vi "EC_Applied_Motion_SXSYSZ_20170419_3ch.vi"() -> ()   [LabVIEW 2015]
uses:
  <vilib>/Utility/file.llb/Read From Spreadsheet File (I64).vi
  <vilib>/Utility/file.llb/Read From Spreadsheet File (string).vi
  <vilib>/Instr/_visa.llb/VISA Configure Serial Port (Instr).vi
  <vilib>/Utility/file.llb/Write To Spreadsheet File (I64).vi
  <vilib>/Utility/file.llb/Write To Spreadsheet File (string).vi
panel:
  in  "Cancel Button":bool
  in  "APX:FZ_JN":bool
  in  "APX:FZ_JP":bool
  in  "APX:FY_JN":bool
  in  "APX:FY_JP":bool
  in  "APX:FX_JN":bool
  in  "APX:FX_JP":bool
  out "Z Velocity MV mm/sec":dbl format="%.3f"
  out "Z Position MV mm":dbl
  out "Y Velocity MV mm/sec":dbl format="%.3f"
  out "Y Position MV mm":dbl
  out "X Velocity MV mm/sec":dbl format="%.3f"
  out "X Position MV mm":dbl
  out "Presets":i32[][](array[numeric])
  in  "stop":bool
  in  "Tab Control 3":enum32{"Status", "Reset"}(tab)
  out "Y in Range":bool
  out "Y Scan":bool
  out "Y in Motion":bool
  out "Y Backlash corr":bool
  out "X  in Range":bool
  out "X Scan":bool
  out "X  in Motion":bool
  out "X Backlash corr":bool
  out "Z in Range":bool
  out "Z Scan":bool
  out "Z in Motion":bool
  out "Z Backlash corr":bool
  out "X Ready":bool
  out "Y Ready":bool
  out "Z Ready":bool
  in  "Reset Y Position mm":dbl
  out "Reset Y Motor Steps":i32
  in  "Reset X Position mm":dbl
  out "Reset X Motor Steps":i32
  in  "Reset Z Position mm":dbl
  out "Reset Z Motor Steps":i32
  in  "Reset":bool
  in  "Tab Control 2":enum32{"mm", "step"}(tab)
  in  "X Scan Length SP mm":dbl
  in  "X Scan Velocity SP mm/sec":dbl
  in  "X Scan set":bool
  in  "Y Scan Length SP mm":dbl
  in  "Y Scan Velocity SP mm/sec":dbl
  in  "Y Scan set":bool
  in  "Z Scan Length SP mm":dbl
  in  "Z Scan Velocity SP mm/sec":dbl
  in  "Z Scan set":bool
  in  "X Scan Velocity SP steps/sec":i32=1 min=1 max=102400 step=1
  in  "X Scan Length SP steps":i32 min=-500000 max=500000 step=100
  out "X Scan length MV mm":dbl
  out "X Scan velocity MV mm/sec":dbl format="%#_6f"
  in  "Y Scan Velocity SP steps/sec":i32=1 min=1 max=102400 step=1
  in  "Y Scan Length SP steps":i32 min=-1000000 max=0 step=100
  out "Y Scan length MV mm":dbl
  out "Y Scan velocity MV mm/sec":dbl format="%#_6f"
  in  "Z Scan Velocity SP steps/sec":i32=1 min=1 max=102400 step=1
  in  "Z Scan Length SP steps":i32 min=-204724 max=102195276 step=100
  out "Z Scan length MV mm":dbl
  out "Z Scan velocity MV mm/sec":dbl format="%#_6f"
  out "atan Y/Z":dbl
  in  "Tab Control":enum32{"mm", "preset", "step"}(tab)
  in  "X Position SP mm":dbl
  in  "X Velocity SP mm/sec":dbl=0.01
  in  "X Move Set":bool
  in  "Y Move Set":bool
  in  "Y Position SP mm":dbl
  in  "Y Velocity SP mm/sec":dbl=0.01
  in  "Z Position SP mm":dbl
  in  "Z Velocity SP mm/sec":dbl=0.05
  in  "Z Move Set":bool
  in  "Add Button":bool
  in  "String":string
  in  "Delete Button":bool
  in  "Preset positions":i32(ring) items=["ZERO", "Default", "CDOSE", "QMS", "test", "test2", "test3"]
  in  "Set Button":bool
  in  "X Velocity SP step/sec":i32 min=1 max=100
  in  "Y Velocity SP step/sec":i32 min=1 max=100
  in  "Z Velocity SP step/sec":i32 min=1 max=50
  in  "Y Step SP":i32=-20000 min=-800000 max=800000 step=500
  in  "X Step SP":i32=-20000 min=-750000 max=750000 step=500
  in  "Z Step SP":i32=-20000 min=-3000 max=102400000 step=500
  out "X Step PV":i32 max=2000
  out "Y Step PV":i32 max=2000
  out "Z Step PV":i32 max=2000
  out "R Step PV":i32 max=2000
  out "X Scan Duration":dbl
  out "Y Scan Duration":dbl
  out "Z Scan Duration":dbl
  out "Z COM PORT":refnum<visa-resource-name>="COM5"
  out "Z Backlash steps/sec":i32
  out "Z Backlash":i32
  out "Z Holding Current %":i32
  out "Z Run Current %":i32
  out "Z offset mm":dbl
  out "Z mm/rev":dbl
  out "Z steps/rev":u32
  out "Z  velocity PV step/sec":i32
  out "Z MINPOS":i32=-94296
  out "Z MAXPOS":i32=-34296
  in  "Z Scan OK":bool
  in  "Z Go":bool
  out "Z Position mm PV":dbl
  out "X Position mm PV":dbl
  out "X velocity PV step/sec":i32
  in  "X Scan OK":bool
  in  "X Go":bool
  out "X Backlash steps/sec":i32
  out "X Backlash":i32
  out "X Holding Current %":i32
  out "X Run Current %":i32
  out "X offset mm":dbl
  out "X mm/rev":dbl
  out "X steps/rev":u32
  out "X MAXPOS":i32=-34296
  out "X MINPOS":i32=-94296
  out "X COM PORT":refnum<visa-resource-name>="COM5"
  out "Y Backlash steps/sec":i32
  out "Y Backlash":i32
  out "Y Holding Current %":i32
  out "Y Run Current %":i32
  in  "Scan Cancel":bool
  out "Y Position mm PV":dbl
  out "Y offset mm":dbl
  out "Y mm/rev":dbl
  out "Y steps/rev":u32
  out "Y velocity PV step/sec":i32
  in  "Y Scan OK":bool
  in  "Scan Go":bool
  in  "Stop":bool
  in  "Y Go":bool
  out "Y MINPOS":i32=-94296
  out "Y MAXPOS":i32=-34296
  out "Y COM PORT":refnum<visa-resource-name>="COM5"
  # "APX:FinePos"
  # "Current position"
  # "Goto position"
  # "APX:FX"
  # "FX"
  # "APX:FY"
  # "FY"
  # "FZ"
  # "APX:FZ"
  # "R,L = green"
  # "L"
  # "M"
  # "B"
  # "S"
  # "R"
  # "Preset position"
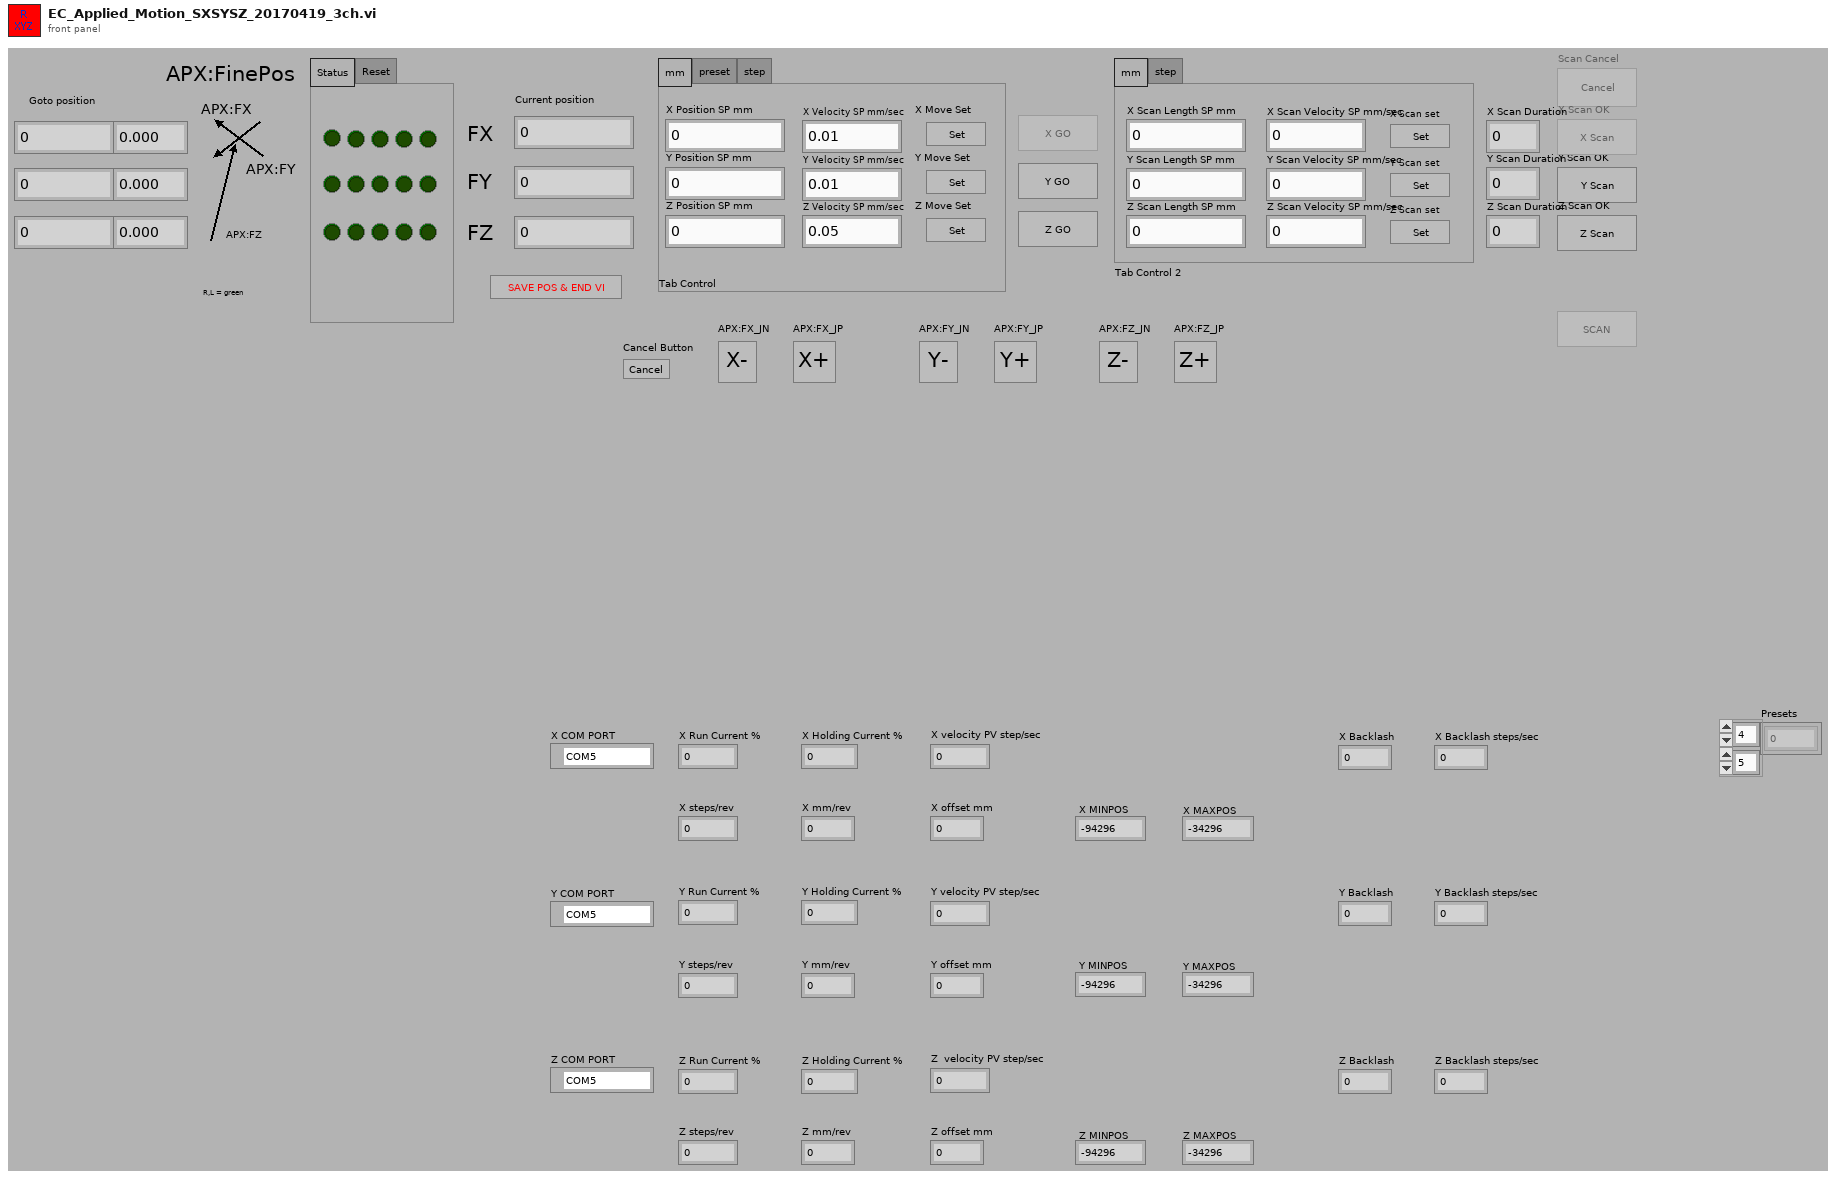
[diagram p1: front panel]
types:
  T1 = enum16{"Power-up Signature", "Accel Rate", "Accel Max", "Bit Rate", "Buffer Status", "Change Current", "Commence Jogging", "Change Jog Speed", "Continue", "Define Address", "Distance for FC,FM,FO,FY", "Decel Rate", "Distance or Position", "Define Limits", "Encoder Deadband", "Encoder Function", "Encoder Position", "Encoder Ratio", "Feed to Length with Speed Change", "Feed to Length", "Feed to Sensor with Mask Dist", "Feed to Length & Set Output", "Feed to Position", "Feed to Sensor", "Feed to Sensor w/safety", "Follow Handwheel", "Immediate Distance?", "Immediate Encoder?", "Immediate Low Output", "Immediate High Output", "Immediate Position?", "Input Status?", "Jog Accel/Decel", "Jog Disable", "Jog Enable", "Jog Speed", "Motor Disable", "Motor Enable", "Microstep Resolution", "Power up Current", "Power up Mode", "Pause", "Request Status", "Revision Level?", "Seek Home", "Stop Jogging", "Stop & Kill Buffer", "Set Output", "Set ABS Position", "Send String", "Stop", "Velocity for Speed Change", "Velocity Setting", "Wait for Input", "Wait Time"}
  T2 = enum8{"Enabled", "Disabled", "Disabled and Grayed Out"}
  T3 = cluster{"first row[0]":i64, "first row[1]":i64, "first row[2]":i64, "first row[3]":i64, "first row[4]":i64, "first row[5]":i64, "first row[6]":i64, "first row[7]":i64, "first row[8]":i64}
  T4 = cluster{"Value[0]":i32, "Value[1]":i32, "Value[2]":i32, "Value[3]":i32, "Value[4]":i32, "Value[5]":i32, "Value[6]":i32, "Value[7]":i32, "Value[8]":i32}
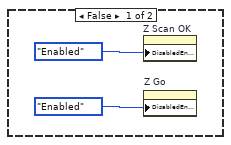
[diagram p5: hidden frame]
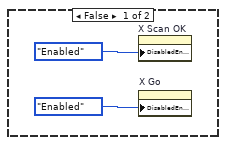
[diagram p9: hidden frame]
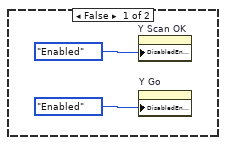
[diagram p13: hidden frame]
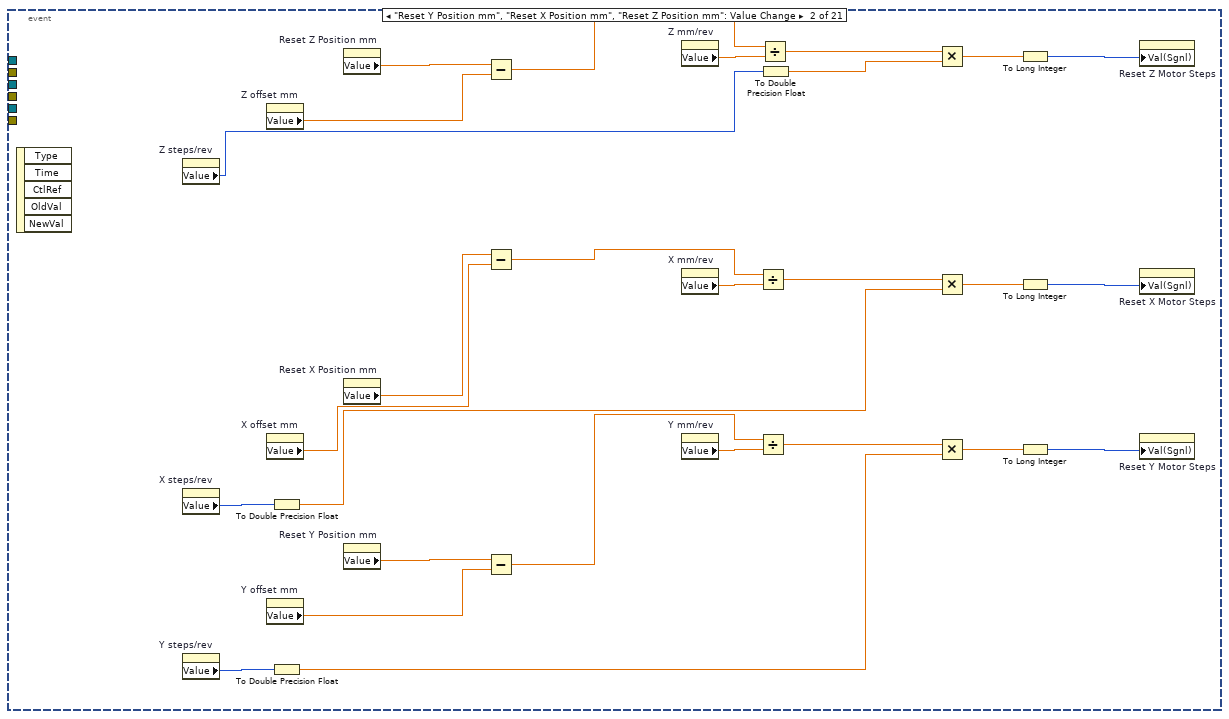
[diagram p17: hidden frame]
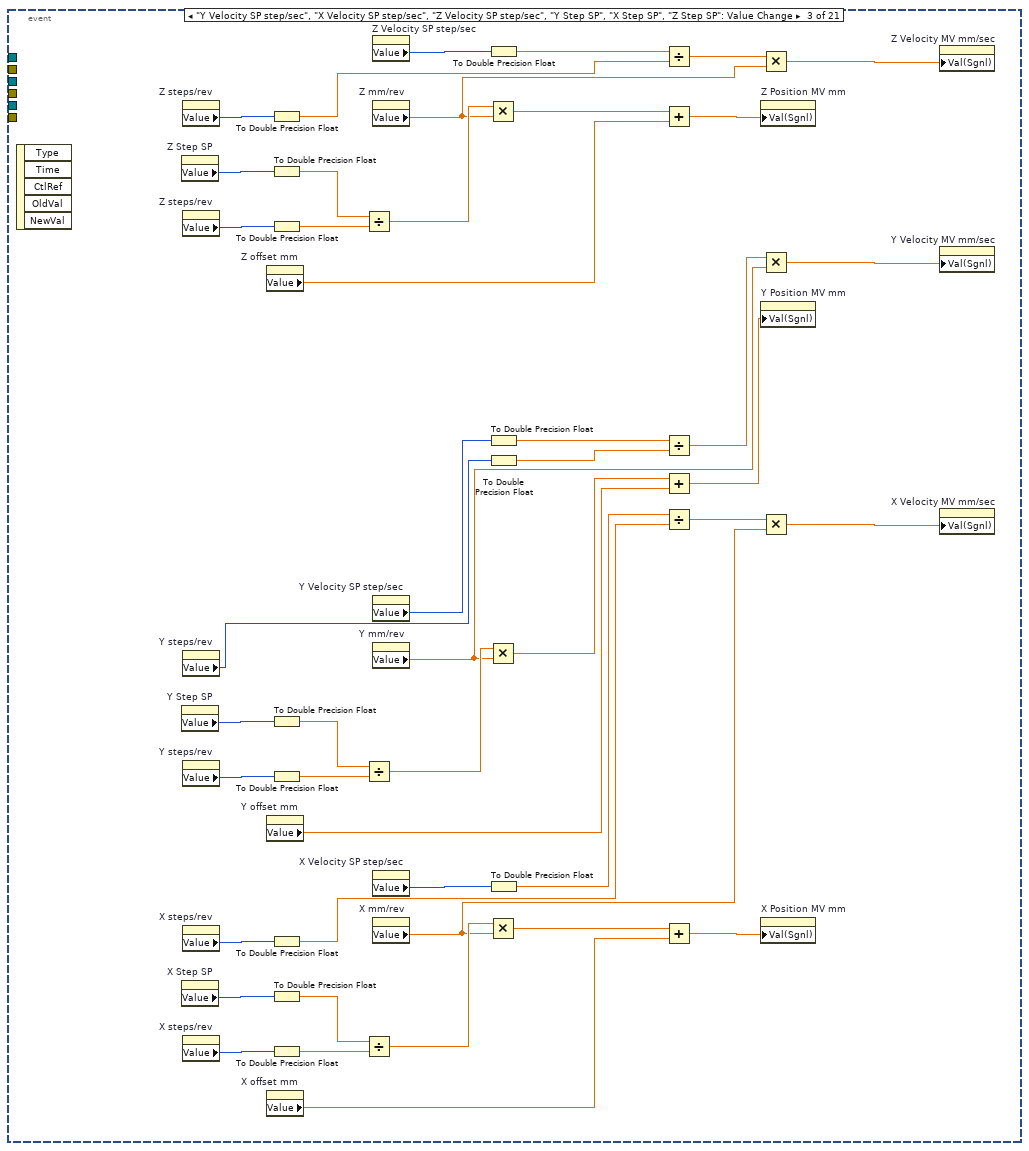
[diagram p18: hidden frame]
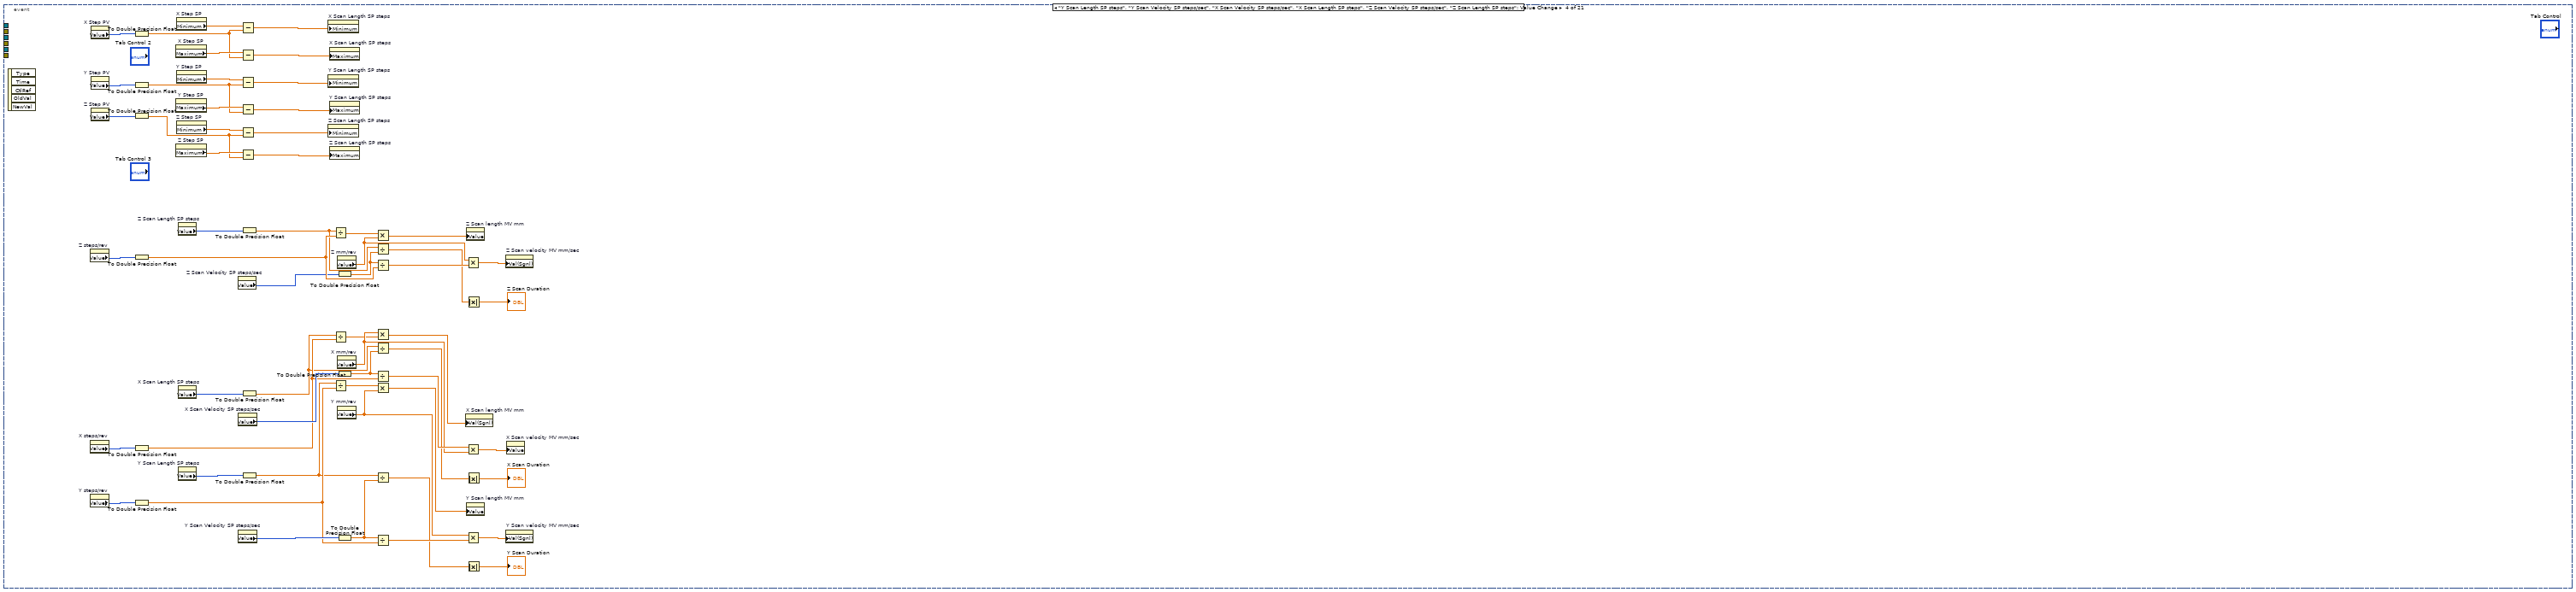
[diagram p19: hidden frame]
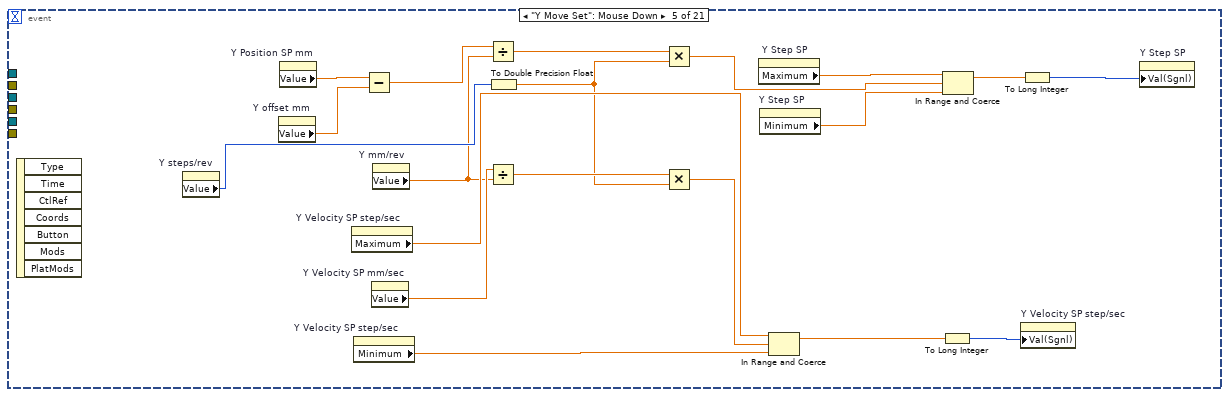
[diagram p20: hidden frame]
diagram:
  (unwired) FALSE
  w19 = 0 ("dimension size")
  n1 = flat-sequence {
    tunnel: [w78] -> w5
    tunnel: [w77] -> w4
    tunnel: w5 -> [w92]
    tunnel: w4 -> [w91]
    tunnel: [w90] -> w3
    tunnel: [w89] -> w2
    tunnel: [w100] -> w49
    tunnel: [w99] -> w48
    tunnel: w3 -> [w102]
    tunnel: w2 -> [w101]
    tunnel: w49 -> [w117]
    tunnel: w48 -> [w116]
    tunnel: [w118] -> w47
    tunnel: [w119] -> w46
    tunnel: [w120] -> w1
    tunnel: [w131] -> w44
    tunnel: [w132] -> w45
    tunnel: w47 -> [w132]
    tunnel: w46 -> [w131]
    tunnel: w1 -> [w129]
    frame #0 {
      "Z Run Current %" <- 100 ("Z Run Current %")
      "Z Holding Current %" <- 50 ("Z Holding Current %")
    }
    frame #1 {
      "Z Backlash steps/sec" <- 1000 ("Z Backlash steps/sec")
      "Z Backlash" <- -2500 ("Z Backlash")
    }
    frame #2 {
      w68 = 2.54 ("Z mm/rev")
      w67 = u32 20000 ("step/rev")
      w69 = 50 ("Value (Signaling)")
      n2 = property on="Z Velocity SP step/sec" class="DigNum (strict)"("Minimum"=1.0 ("Data Entry Limits:Minimum")) -> ()  [unwired: 2 in, 2 out]
      n3 = property on="Z Scan Velocity SP mm/sec" class="DigNum (strict)"("Val(Sgnl)"=0.05 ("Value (Signaling)")) -> ()  [unwired: 2 in, 2 out]
      n4 = property on="Z Velocity SP step/sec" class="DigNum (strict)"("Val(Sgnl)"=w69) -> ()  [unwired: 2 in, 2 out]
      n5 = To Double Precision Float(number=w69) -> (double precision float=w73:dbl)
      n6 = property on="Z Velocity SP step/sec" class="DigNum (strict)"("Maximum"=w73) -> ()  [unwired: 2 in, 2 out]
      n7 = To Double Precision Float(number=w67) -> (double precision float=w72:dbl)
      n8 = Divide(x=w73, y=w72) -> (x/y=w70:dbl)
      n9 = Multiply(x=w70, y=w68) -> (x*y=w71:dbl)
      n10 = property on="Z Velocity SP mm/sec" class="DigNum (strict)"("Val(Sgnl)"=w71) -> ()  [unwired: 2 in, 2 out]
      "Z mm/rev" <- w68
      "Z steps/rev" <- w67
    }
    frame #3 {
      w75 = -3000 ("lower limit")
      w74 = 102400000 ("upper limit")
      n11 = property on="Z Step SP" class="DigNum (strict)"("Minimum"=w75) -> ()  [unwired: 2 in, 2 out]
      n12 = property on="Z Step SP" class="DigNum (strict)"("Maximum"=w74) -> ()  [unwired: 2 in, 2 out]
      "Z offset mm" <- 0.0 ("Z offset mm")
      "Z MINPOS" <- w75
      "Z MAXPOS" <- w74
    }
    frame #4 {
      w85 = refnum<visa-resource-name> "COM23" ("COM PORT")
      w83 = u16 0 items=["None", "XON/XOFF", "RTS/CTS", "XON/XOFF & RTS/CTS", "DTR/DSR", "XON/XOFF & DTR/DSR"] ("flow control (0:none)")
      w82 = u16 10 items=["1.0"=10, "1.5"=15, "2.0"=20] ("stop bits (10: 1 bit)")
      # "Stop bits"
      n13 = call-poly "VISA Configure Serial Port"("VISA resource name"=w85, "timeout (10sec)"=u32 10000, "baud rate (9600)"=u32 9600, "data bits (8)"=u16 8, "parity (0:none)"=enum16{"None", "Odd", "Even", "Mark", "Space"}."None", "stop bits (10: 1 bit)"=w82, "flow control (0:none)"=w83) -> ("VISA resource name out"=w78:refnum<visa-resource-name>, "error out"=w77:errorcluster)  [unwired: 7 in]
      "Z COM PORT" <- w85
    }
    frame #5 {
      # "Run Current %"
      n14 = property on="Z Run Current %" class="DigNum (strict)"() -> ("Value"=w93:i32)  [unwired: 2 in, 2 out]
      n15 = Divide(x=w93, y=100) -> (x/y=w94:dbl)
      n16 = Multiply(x=w94, y=3.5) -> (x*y=w88:dbl)
      n17 = Number To Fractional String(number=w88) -> (F-format string=w95:string)  [unwired: 3 in]
      n18 = call "Applied Send Command.vi"("error in (no error)"=w91, "Extra"=w95, "Command"=T1."Change Current", "VISA resource name"=w92) -> ("error out"=w89:errorcluster, "VISA resource name out"=w90:refnum<visa-resource-name>)  [unwired: 3 in, 1 out]
    }
    frame #6 {
      # "VELOCITY"
      n19 = property on="Z steps/rev" class="DigNum (strict)"() -> ("Value"=w98:u32)  [unwired: 2 in, 2 out]
      n20 = property on="Z Velocity SP step/sec" class="DigNum (strict)"() -> ("Value"=w97:i32)  [unwired: 2 in, 2 out]
      n21 = Divide(x=w97, y=w98) -> (x/y=w105:dbl)
      n22 = Number To Fractional String(number=w105) -> (F-format string=w107:string)  [unwired: 3 in]
      n23 = call "Applied Send Command.vi"("error in (no error)"=w101, "Extra"=w107, "Command"=T1."Velocity Setting", "VISA resource name"=w102) -> ("error out"=w108:errorcluster, "VISA resource name out"=w115:refnum<visa-resource-name>)  [unwired: 3 in, 1 out]
      n24 = call "Time Delay2"("error in (no error)"=w108, "Delay Time (s)"=0.1) -> ("error out"=w113:errorcluster)  [unwired: 9 in]
      n25 = call "Applied Send Command.vi"("error in (no error)"=w113, "Extra"="", "Command"=T1."Velocity Setting", "VISA resource name"=w115) -> ("error out"=w99:errorcluster, "read buffer"=w111:string, "VISA resource name out"=w100:refnum<visa-resource-name>)  [unwired: 3 in]
      n26 = Fract/Exp String To Number(string=w111, offset=3) -> (number=w106:dbl)  [unwired: 2 in, 1 out]
      n27 = Multiply(x=w106, y=w98) -> (x*y=w103:dbl)
      n28 = property on="Z  velocity PV step/sec" class="DigNum (strict)"("Val(Sgnl)"=w103) -> ()  [unwired: 2 in, 2 out]
    }
    frame #7 {
      # "GET CURRENT POSITION"
      n29 = call "Applied Send Command.vi"("error in (no error)"=w116, "Extra"="", "Command"=T1."Immediate Position?", "VISA resource name"=w117) -> ("error out"=w122:errorcluster, "read buffer"=w124:string, "VISA resource name out"=w118:refnum<visa-resource-name>)  [unwired: 3 in]
      n30 = call "Time Delay8"("error in (no error)"=w122, "Delay Time (s)"=0.1) -> ("error out"=w119:errorcluster)  [unwired: 9 in]
      n31 = Hexadecimal String To Number(string=w124, offset=3) -> (number=w120:u32)  [unwired: 1 in, 1 out]
    }
    frame #8 {
      n32 = property on="Z Step SP" class="DigNum (strict)"() -> ("Maximum"=w128:dbl)  [unwired: 2 in, 2 out]
      n33 = property on="Z Step SP" class="DigNum (strict)"() -> ("Minimum"=w127:dbl)  [unwired: 2 in, 2 out]
      n34 = property on="Z Step SP" class="DigNum (strict)"("Val(Sgnl)"=w129) -> ()  [unwired: 2 in, 2 out]
      n35 = In Range and Coerce(upper limit=w128, x=w129, lower limit=w127) -> (In Range?=w130:bool)  [unwired: 1 out]
      n36 = property on="Z in Range" class="Bool (strict)"("Val(Sgnl)"=w130) -> ()  [unwired: 2 in, 2 out]
    }
  }
  n37 = flat-sequence {
    frame #0 {
      n38 = property on="X Scan" class="Bool (strict)"("Val(Sgnl)"=FALSE ("Value (Signaling)")) -> ()  [unwired: 2 in, 2 out]
      n39 = property on="Y Scan" class="Bool (strict)"("Val(Sgnl)"=FALSE ("Value (Signaling)")) -> ()  [unwired: 2 in, 2 out]
      n40 = property on="Z Scan" class="Bool (strict)"("Val(Sgnl)"=FALSE ("Value (Signaling)")) -> ()  [unwired: 2 in, 2 out]
      n41 = property on="Scan Go" class="Bool"("DisabledEnum"=T2."Disabled and Grayed Out" ("Disabled")) -> ()  [unwired: 2 in, 2 out]
      n42 = property on="Scan Cancel" class="Bool"("DisabledEnum"=T2."Disabled and Grayed Out" ("Disabled")) -> ()  [unwired: 2 in, 2 out]
    }
    frame #1 {
      n43 = property on="Y Backlash corr" class="Bool (strict)"("Val(Sgnl)"=FALSE ("Value (Signaling)")) -> ()  [unwired: 2 in, 2 out]
      n44 = property on="X Backlash corr" class="Bool (strict)"("Val(Sgnl)"=FALSE ("Value (Signaling)")) -> ()  [unwired: 2 in, 2 out]
      n45 = property on="Z Backlash corr" class="Bool (strict)"("Val(Sgnl)"=FALSE ("Value (Signaling)")) -> ()  [unwired: 2 in, 2 out]
    }
  }
  n46 = flat-sequence {
    tunnel: [w158] -> w13
    tunnel: [w157] -> w12
    tunnel: w13 -> [w172]
    tunnel: w12 -> [w171]
    tunnel: [w170] -> w11
    tunnel: [w169] -> w10
    tunnel: w11 -> [w180]
    tunnel: w10 -> [w179]
    tunnel: [w178] -> w9
    tunnel: [w177] -> w8
    tunnel: [w197] -> w53
    tunnel: w9 -> [w200]
    tunnel: w8 -> [w199]
    tunnel: [w198] -> w7
    tunnel: [w196] -> w6
    tunnel: [w209] -> w59
    tunnel: [w212] -> w60
    tunnel: w53 -> [w209]
    tunnel: w7 -> [w212]
    tunnel: w6 -> [w210]
    frame #0 {
      "Y Run Current %" <- 100 ("Run Current %")
      "Y Holding Current %" <- 50 ("Holding Current %")
    }
    frame #1 {
      "Y Backlash" <- 5000 ("Backlash2")
      "Y Backlash steps/sec" <- 10000 ("Value (Signaling)")
    }
    frame #2 {
      w148 = 0.21167 ("MM/rev")
      w151 = u32 20000 ("step/rev")
      w146 = 100 ("Value (Signaling)")
      n47 = property on="Y Velocity SP step/sec" class="DigNum (strict)"("Minimum"=1.0 ("Data Entry Limits:Minimum")) -> ()  [unwired: 2 in, 2 out]
      n48 = property on="Y Scan Velocity SP mm/sec" class="DigNum (strict)"("Val(Sgnl)"=0.01 ("Value (Signaling)")) -> ()  [unwired: 2 in, 2 out]
      n49 = property on="Y Velocity SP step/sec" class="DigNum (strict)"("Val(Sgnl)"=w146) -> ()  [unwired: 2 in, 2 out]
      n50 = To Double Precision Float(number=w146) -> (double precision float=w152:dbl)
      n51 = property on="Y Velocity SP step/sec" class="DigNum (strict)"("Maximum"=w152) -> ()  [unwired: 2 in, 2 out]
      n52 = To Double Precision Float(number=w151) -> (double precision float=w150:dbl)
      n53 = Divide(x=w152, y=w150) -> (x/y=w147:dbl)
      n54 = Multiply(x=w147, y=w148) -> (x*y=w149:dbl)
      n55 = property on="Y Velocity SP mm/sec" class="DigNum (strict)"("Val(Sgnl)"=w149) -> ()  [unwired: 2 in, 2 out]
      "Y steps/rev" <- w151
      "Y mm/rev" <- w148
    }
    frame #3 {
      w155 = -800000 ("lower limit")
      w156 = 800000 ("upper limit")
      n56 = property on="Y Step SP" class="DigNum (strict)"("Minimum"=w155) -> ()  [unwired: 2 in, 2 out]
      n57 = property on="Y Step SP" class="DigNum (strict)"("Maximum"=w156) -> ()  [unwired: 2 in, 2 out]
      "Y MAXPOS" <- w156
      "Y MINPOS" <- w155
      "Y offset mm" <- 0.0 ("offset")
    }
    frame #4 {
      w165 = refnum<visa-resource-name> "COM22" ("COM PORT")
      w163 = u16 0 items=["None", "XON/XOFF", "RTS/CTS", "XON/XOFF & RTS/CTS", "DTR/DSR", "XON/XOFF & DTR/DSR"] ("flow control (0:none)")
      w162 = u16 10 items=["1.0"=10, "1.5"=15, "2.0"=20] ("stop bits (10: 1 bit)")
      # "Stop bits"
      n58 = call-poly "VISA Configure Serial Port"("VISA resource name"=w165, "timeout (10sec)"=u32 10000, "baud rate (9600)"=u32 9600, "data bits (8)"=u16 8, "parity (0:none)"=enum16{"None", "Odd", "Even", "Mark", "Space"}."None", "stop bits (10: 1 bit)"=w162, "flow control (0:none)"=w163) -> ("VISA resource name out"=w158:refnum<visa-resource-name>, "error out"=w157:errorcluster)  [unwired: 7 in]
      "Y COM PORT" <- w165
    }
    frame #5 {
      n59 = property on="Y Run Current %" class="DigNum (strict)"() -> ("Value"=w173:i32)  [unwired: 2 in, 2 out]
      n60 = Divide(x=w173, y=100) -> (x/y=w174:dbl)
      n61 = Multiply(x=w174, y=3.5) -> (x*y=w168:dbl)
      n62 = Number To Fractional String(number=w168) -> (F-format string=w175:string)  [unwired: 3 in]
      n63 = call "Applied Send Command.vi"("error in (no error)"=w171, "Extra"=w175, "Command"=T1."Change Current", "VISA resource name"=w172) -> ("error out"=w169:errorcluster, "VISA resource name out"=w170:refnum<visa-resource-name>)  [unwired: 3 in, 1 out]
    }
    frame #6 {
      # "VELOCITY"
      n64 = property on="Y steps/rev" class="DigNum (strict)"() -> ("Value"=w184:u32)  [unwired: 2 in, 2 out]
      n65 = property on="Y Velocity SP step/sec" class="DigNum (strict)"() -> ("Value"=w181:i32)  [unwired: 2 in, 2 out]
      n66 = Divide(x=w181, y=w184) -> (x/y=w183:dbl)
      n67 = Number To Fractional String(number=w183) -> (F-format string=w187:string)  [unwired: 3 in]
      n68 = call "Applied Send Command.vi"("error in (no error)"=w179, "Extra"=w187, "Command"=T1."Velocity Setting", "VISA resource name"=w180) -> ("error out"=w188:errorcluster, "VISA resource name out"=w195:refnum<visa-resource-name>)  [unwired: 3 in, 1 out]
      n69 = call "Time Delay36"("error in (no error)"=w188, "Delay Time (s)"=0.1) -> ("error out"=w193:errorcluster)  [unwired: 9 in]
      n70 = call "Applied Send Command.vi"("error in (no error)"=w193, "Extra"="", "Command"=T1."Velocity Setting", "VISA resource name"=w195) -> ("error out"=w177:errorcluster, "read buffer"=w191:string, "VISA resource name out"=w178:refnum<visa-resource-name>)  [unwired: 3 in]
      n71 = Fract/Exp String To Number(string=w191, offset=3) -> (number=w186:dbl)  [unwired: 2 in, 1 out]
      n72 = Multiply(x=w186, y=w184) -> (x*y=w185:dbl)
      n73 = property on="Y velocity PV step/sec" class="DigNum (strict)"("Val(Sgnl)"=w185) -> ()  [unwired: 2 in, 2 out]
    }
    frame #7 {
      # "GET CURRENT POSITION"
      n74 = call "Applied Send Command.vi"("error in (no error)"=w199, "Extra"="", "Command"=T1."Immediate Position?", "VISA resource name"=w200) -> ("error out"=w202:errorcluster, "read buffer"=w204:string, "VISA resource name out"=w198:refnum<visa-resource-name>)  [unwired: 3 in]
      n75 = call "Time Delay37"("error in (no error)"=w202, "Delay Time (s)"=0.1) -> ("error out"=w197:errorcluster)  [unwired: 9 in]
      n76 = Hexadecimal String To Number(string=w204, offset=3) -> (number=w196:u32)  [unwired: 1 in, 1 out]
    }
    frame #8 {
      n77 = property on="Y Step SP" class="DigNum (strict)"() -> ("Maximum"=w208:dbl)  [unwired: 2 in, 2 out]
      n78 = property on="Y Step SP" class="DigNum (strict)"() -> ("Minimum"=w207:dbl)  [unwired: 2 in, 2 out]
      n79 = property on="Y Step SP" class="DigNum (strict)"("Val(Sgnl)"=w210) -> ()  [unwired: 2 in, 2 out]
      n80 = In Range and Coerce(upper limit=w208, x=w210, lower limit=w207) -> (In Range?=w211:bool)  [unwired: 1 out]
      n81 = property on="Y in Range" class="Bool (strict)"("Val(Sgnl)"=w211) -> ()  [unwired: 2 in, 2 out]
    }
  }
  n82 = flat-sequence {
    tunnel: [w230] -> w18
    tunnel: [w229] -> w17
    tunnel: w18 -> [w247]
    tunnel: w17 -> [w246]
    tunnel: [w245] -> w16
    tunnel: [w244] -> w15
    tunnel: [w250] -> w58
    tunnel: w16 -> [w258]
    tunnel: w15 -> [w257]
    tunnel: [w251] -> w14
    tunnel: w58 -> [w272]
    tunnel: [w271] -> w52
    tunnel: [w269] -> w51
    tunnel: [w274] -> w50
    tunnel: w14 -> [w273]
    tunnel: [w283] -> w56
    tunnel: [w284] -> w57
    tunnel: w52 -> [w284]
    tunnel: w51 -> [w283]
    tunnel: w50 -> [w279]
    frame #0 {
      "X Run Current %" <- 100 ("Run Current %")
      "X Holding Current %" <- 50 ("Holding Current %")
    }
    frame #1 {
      "X Backlash steps/sec" <- 10000 ("Value (Signaling)")
      "X Backlash" <- 5000 ("Backlash2")
    }
    frame #2 {
      w219 = 0.21167 ("MM/rev")
      w222 = u32 20000 ("step/rev")
      w217 = 100 ("Value (Signaling)")
      n83 = property on="X Velocity SP step/sec" class="DigNum (strict)"("Minimum"=1.0 ("Data Entry Limits:Minimum")) -> ()  [unwired: 2 in, 2 out]
      n84 = property on="X Velocity SP step/sec" class="DigNum (strict)"("Val(Sgnl)"=w217) -> ()  [unwired: 2 in, 2 out]
      n85 = property on="X Scan Velocity SP mm/sec" class="DigNum (strict)"("Val(Sgnl)"=0.01 ("Value (Signaling)")) -> ()  [unwired: 2 in, 2 out]
      n86 = To Double Precision Float(number=w217) -> (double precision float=w223:dbl)
      n87 = property on="X Velocity SP step/sec" class="DigNum (strict)"("Maximum"=w223) -> ()  [unwired: 2 in, 2 out]
      n88 = To Double Precision Float(number=w222) -> (double precision float=w221:dbl)
      n89 = Divide(x=w223, y=w221) -> (x/y=w218:dbl)
      n90 = Multiply(x=w218, y=w219) -> (x*y=w220:dbl)
      n91 = property on="X Velocity SP mm/sec" class="DigNum (strict)"("Val(Sgnl)"=w220) -> ()  [unwired: 2 in, 2 out]
      "X steps/rev" <- w222
      "X mm/rev" <- w219
    }
    frame #3 {
      w228 = -750000 ("lower limit")
      w227 = 750000 ("upper limit")
      n92 = property on="X Step SP" class="DigNum (strict)"("Minimum"=w228) -> ()  [unwired: 2 in, 2 out]
      n93 = property on="X Step SP" class="DigNum (strict)"("Maximum"=w227) -> ()  [unwired: 2 in, 2 out]
      "X offset mm" <- 0.0 ("offset")
      "X MAXPOS" <- w227
      "X MINPOS" <- w228
    }
    frame #4 {
      w237 = refnum<visa-resource-name> "COM21" ("COM PORT")
      w235 = u16 0 items=["None", "XON/XOFF", "RTS/CTS", "XON/XOFF & RTS/CTS", "DTR/DSR", "XON/XOFF & DTR/DSR"] ("flow control (0:none)")
      w234 = u16 10 items=["1.0"=10, "1.5"=15, "2.0"=20] ("stop bits (10: 1 bit)")
      # "Stop bits"
      n94 = call-poly "VISA Configure Serial Port"("VISA resource name"=w237, "timeout (10sec)"=u32 10000, "baud rate (9600)"=u32 9600, "data bits (8)"=u16 8, "parity (0:none)"=enum16{"None", "Odd", "Even", "Mark", "Space"}."None", "stop bits (10: 1 bit)"=w234, "flow control (0:none)"=w235) -> ("VISA resource name out"=w230:refnum<visa-resource-name>, "error out"=w229:errorcluster)  [unwired: 7 in]
      "X COM PORT" <- w237
    }
    frame #5 {
      n95 = property on="X Run Current" class="DigNum (strict)"() -> ("Value"=w242:i32)  [unwired: 2 in, 2 out]
      n96 = Divide(x=w242, y=100) -> (x/y=w239:dbl)
      n97 = Multiply(x=3.5 ("y"), y=w239) -> (x*y=w241:dbl)
      n98 = Number To Fractional String(number=w241) -> (F-format string=w243:string)  [unwired: 3 in]
      n99 = call "Applied Send Command.vi"("error in (no error)"=w246, "Extra"=w243, "Command"=T1."Change Current", "VISA resource name"=w247) -> ("error out"=w245:errorcluster, "VISA resource name out"=w244:refnum<visa-resource-name>)  [unwired: 3 in, 1 out]
    }
    frame #6 {
      # "VELOCITY"
      n100 = property on="X steps/rev" class="DigNum (strict)"() -> ("Value"=w253:u32)  [unwired: 2 in, 2 out]
      n101 = property on="X Velocity SP step/sec" class="DigNum (strict)"() -> ("Value"=w254:i32)  [unwired: 2 in, 2 out]
      n102 = Divide(x=w254, y=w253) -> (x/y=w252:dbl)
      n103 = Number To Fractional String(number=w252) -> (F-format string=w259:string)  [unwired: 3 in]
      n104 = call "Applied Send Command.vi"("error in (no error)"=w258, "Extra"=w259, "Command"=T1."Velocity Setting", "VISA resource name"=w257) -> ("error out"=w260:errorcluster, "VISA resource name out"=w267:refnum<visa-resource-name>)  [unwired: 3 in, 1 out]
      n105 = call "Time Delay30"("error in (no error)"=w260, "Delay Time (s)"=0.1) -> ("error out"=w265:errorcluster)  [unwired: 9 in]
      n106 = call "Applied Send Command.vi"("error in (no error)"=w265, "Extra"="", "Command"=T1."Velocity Setting", "VISA resource name"=w267) -> ("error out"=w250:errorcluster, "read buffer"=w263:string, "VISA resource name out"=w251:refnum<visa-resource-name>)  [unwired: 3 in]
      n107 = Fract/Exp String To Number(string=w263, offset=3) -> (number=w256:dbl)  [unwired: 2 in, 1 out]
      n108 = Multiply(x=w256, y=w253) -> (x*y=w255:dbl)
      n109 = property on="X velocity PV step/sec" class="DigNum (strict)"("Val(Sgnl)"=w255) -> ()  [unwired: 2 in, 2 out]
    }
    frame #7 {
      # "GET CURRENT POSITION"
      n110 = call "Applied Send Command.vi"("error in (no error)"=w272, "Extra"="", "Command"=T1."Immediate Position?", "VISA resource name"=w273) -> ("error out"=w270:errorcluster, "read buffer"=w276:string, "VISA resource name out"=w271:refnum<visa-resource-name>)  [unwired: 3 in]
      n111 = call "Time Delay13"("error in (no error)"=w270, "Delay Time (s)"=0.1) -> ("error out"=w269:errorcluster)  [unwired: 9 in]
      n112 = Hexadecimal String To Number(string=w276, offset=3) -> (number=w274:u32)  [unwired: 1 in, 1 out]
    }
    frame #8 {
      n113 = property on="X Step SP" class="DigNum (strict)"() -> ("Maximum"=w282:dbl)  [unwired: 2 in, 2 out]
      n114 = property on="X Step SP" class="DigNum (strict)"() -> ("Minimum"=w281:dbl)  [unwired: 2 in, 2 out]
      n115 = property on="X Step SP" class="DigNum (strict)"("Val(Sgnl)"=w279) -> ()  [unwired: 2 in, 2 out]
      n116 = In Range and Coerce(upper limit=w282, x=w279, lower limit=w281) -> (In Range?=w280:bool)  [unwired: 1 out]
      n117 = property on="X  in Range" class="Bool (strict)"("Val(Sgnl)"=w280) -> ()  [unwired: 2 in, 2 out]
    }
  }
  n118 = call-poly <vilib>:"Read From Spreadsheet File.vi"("file path (dialog if empty)"=path "S:/SSE/SCL2/POS.TXT") -> ("first row"=w36:i64[])  [unwired: 6 in, 4 out]
  n119 = call-poly <vilib>:"Read From Spreadsheet File.vi"("file path (dialog if empty)"=path "S:/SSE/SCL2/PRESET.TXT") -> ("all rows"=w25:string[][])  [unwired: 6 in, 4 out]
  n120 = Array To Cluster(array=w36) -> (cluster=w35:T3)
  n121 = Transpose 2D Array(2D array=w25) -> (transposed array=w26:string[][])
  n122 = Unbundle(w35) -> ("first row[0]"=w33:i64, "first row[1]"=w32:i64, "first row[2]"=w31:i64)  [unwired: 6 out]
  n123 = Delete From Array(array=w26, index (row)=0) -> (deleted portion=w27:string[], array with subset deleted=w29:string[][])  [unwired: 2 in]
  n124 = property on="Reset X Motor Steps" class="DigNum (strict)"("Val(Sgnl)"=w33) -> ()  [unwired: 2 in, 2 out]
  n125 = property on="Reset Y Motor Steps" class="DigNum (strict)"("Val(Sgnl)"=w32) -> ()  [unwired: 2 in, 2 out]
  n126 = property on="Reset Z Motor Steps" class="DigNum (strict)"("Val(Sgnl)"=w31) -> ()  [unwired: 2 in, 2 out]
  n127 = property on="Preset positions" class="Ring (strict)"("Strings []"=w27) -> ()  [unwired: 2 in, 2 out]
  n128 = Transpose 2D Array(2D array=w29) -> (transposed array=w30:string[][])
  n129 = Decimal String To Number(string=w30) -> (number=w28:i32[][])  [unwired: 2 in, 1 out]
  n130 = Initialize Array(w19, w19, 4 ("dimension size")) -> (w22:i32[][])
  n131 = Build Array (concatenate)(w22, w28) -> (→"Presets":i32[][])
  n132 = while {
    tunnel: w60 -> [w301]
    tunnel: w59 -> [w304]
    tunnel: [w305] -> w40
    tunnel: [w303] -> w41
    tunnel: w57 -> [w300]
    tunnel: w56 -> [w299]
    tunnel: [w298] -> w55
    tunnel: [w297] -> w54
    tunnel: w45 -> [w296]
    tunnel: w44 -> [w295]
    tunnel: [w294] -> w43
    tunnel: [w293] -> w42
    tunnel: [w292] -> _
    tunnel: [w291] -> _
    stop <- "stop" stop-if-true
    n133 = flat-sequence {
      frame #0 {
      }
      frame #1 {
      }
    }
    n134 = flat-sequence {
      frame #0 {
      }
      frame #1 {
      }
    }
    n135 = property on="Preset positions" class="Ring (strict)"() -> ("Strings []"=w287:string[])  [unwired: 2 in, 2 out]
    n136 = event shown="[0] Timeout" {
      selector: _ -> [_ _ _ _ _ _ _ _ _ _ _ _ _ _ _ _ _ _ _ _ _]
      dyn-events: _ -> [_ _ _ _ _ _ _ _ _ _ _ _ _ _ _ _ _ _ _ _ _]
      timeout: 200 -> [_ _ _ _ _ _ _ _ _ _ _ _ _ _ _ _ _ _ _ _ _]
      tunnel: w304 -> [w398 _ _ _ _ _ _ _ _ _ w960 _ _ _ w1190 _ w1257 w1269 w1302 w1368 w1478]
      tunnel: [w397 _ _ _ _ _ _ _ _ _ w966 _ _ _ w1188 _ w1257 w1267 w1304 w1364 w1476] -> w305
      tunnel: w301 -> [w355 _ _ _ _ _ _ _ _ _ w961 _ _ _ w1189 _ w1258 w1270 w1303 w1369 w1479]
      tunnel: [w396 _ _ _ _ _ _ _ _ _ w967 _ _ _ w1185 _ w1258 w1268 w1305 w1365 w1477] -> w303
      tunnel: w300 -> [w354 _ _ _ _ _ _ _ _ _ _ _ w1091 w1151 _ _ _ w1264 w1295 w1371 w1475]
      tunnel: w299 -> [w373 _ _ _ _ _ _ _ _ _ _ _ w1090 w1150 _ _ _ w1263 w1294 w1370 w1474]
      tunnel: [w372 _ _ _ _ _ _ _ _ _ _ _ w1089 w1149 _ _ _ w1266 w1293 w1361 w1473] -> w298
      tunnel: [w371 _ _ _ _ _ _ _ _ _ _ _ w1088 w1148 _ _ _ w1265 w1292 w1360 w1472] -> w297
      tunnel: w296 -> [w356 _ _ _ _ _ _ _ _ _ _ w1023 _ _ _ w1223 _ w1262 w1289 w1367 w1471]
      tunnel: w295 -> [w359 _ _ _ _ _ _ _ _ _ _ w1022 _ _ _ w1222 _ w1261 w1288 w1366 w1470]
      tunnel: [w358 _ _ _ _ _ _ _ _ _ _ w1020 _ _ _ w1220 _ w1260 w1287 w1363 _] -> w294
      tunnel: [w357 _ _ _ _ _ _ _ _ _ _ w1021 _ _ _ w1221 _ w1259 w1286 w1362 _] -> w293
      tunnel: [_ _ _ _ _ _ _ _ _ _ _ _ _ _ _ _ _ _ _ _ w1469] -> w292
      tunnel: [_ _ _ _ _ _ _ _ _ _ _ _ _ _ _ _ _ _ _ _ w1468] -> w291
      event Timeout {
        n137 = event-data() -> ()  [unwired: 1 in, 2 out]
        n138 = property on="X Step SP" class="DigNum (strict)"() -> ("Maximum"=w338:dbl)  [unwired: 2 in, 2 out]
        n139 = property on="Y Step SP" class="DigNum (strict)"() -> ("Maximum"=w343:dbl)  [unwired: 2 in, 2 out]
        n140 = property on="X Step SP" class="DigNum (strict)"() -> ("Minimum"=w339:dbl)  [unwired: 2 in, 2 out]
        n141 = property on="Y Step SP" class="DigNum (strict)"() -> ("Minimum"=w342:dbl)  [unwired: 2 in, 2 out]
        n142 = flat-sequence {
          tunnel: [w407] -> w370
          tunnel: [w420] -> w369
          tunnel: [w430] -> w368
          tunnel: [w400] -> w367
          tunnel: w356 -> [w415]
          tunnel: w359 -> [w416]
          tunnel: w370 -> [w440]
          tunnel: [w440] -> w366
          tunnel: w369 -> [w439]
          tunnel: [w439] -> w365
          tunnel: w368 -> [w438]
          tunnel: [w438] -> w364
          tunnel: w367 -> [w435]
          tunnel: [w435] -> w363
          tunnel: w366 -> [w447]
          tunnel: [w448] -> w362
          tunnel: w365 -> [w450]
          tunnel: [w449] -> w361
          tunnel: w364 -> [w446]
          tunnel: [w445] -> w360
          tunnel: w363 -> [w445]
          tunnel: w362 -> [w460]
          tunnel: w361 -> [w461]
          tunnel: w360 -> [w462]
          tunnel: [w459] -> w357
          tunnel: [w458] -> w358
          frame #0 {
            w419 = 0.2 ("Delay Time (s)")
            n143 = property on="Z Step SP" class="DigNum (strict)"() -> ("Maximum"=w432:dbl)  [unwired: 2 in, 2 out]
            n144 = property on="Z Step SP" class="DigNum (strict)"() -> ("Minimum"=w434:dbl)  [unwired: 2 in, 2 out]
            n145 = property on="Z steps/rev" class="DigNum (strict)"() -> ("Value"=w428:u32)  [unwired: 2 in, 2 out]
            n146 = property on="Z offset mm" class="DigNum (strict)"() -> ("Value"=w424:dbl)  [unwired: 2 in, 2 out]
            n147 = To Long Integer(number=w432) -> (32bit integer=w431:i32)
            n148 = To Long Integer(number=w434) -> (32bit integer=w433:i32)
            n149 = To Double Precision Float(number=w428) -> (double precision float=w429:dbl)
            n150 = call "Applied Send Command.vi"("error in (no error)"=w416, "Command"=T1."Immediate Position?", "VISA resource name"=w415) -> ("error out"=w414:errorcluster, "read buffer"=w411:string, "VISA resource name out"=w409:refnum<visa-resource-name>)  [unwired: 4 in]
            n151 = call "Time Delay17"("error in (no error)"=w414, "Delay Time (s)"=w419) -> ("error out"=w399:errorcluster)  [unwired: 9 in]
            n152 = Hexadecimal String To Number(string=w411, offset=3) -> (number=w412:u32)  [unwired: 1 in, 1 out]
            n153 = To Long Integer(number=w412) -> (32bit integer=w422:i32)
            n154 = call "Applied Send Command.vi"("error in (no error)"=w399, "Command"=T1."Request Status", "VISA resource name"=w409) -> ("error out"=w408:errorcluster, "read buffer"=w404:string, "VISA resource name out"=w407:refnum<visa-resource-name>)  [unwired: 4 in]
            n155 = property on="Z Step PV" class="DigNum (strict)"("Val(Sgnl)"=w422) -> ()  [unwired: 2 in, 2 out]
            n156 = call "Time Delay16"("error in (no error)"=w408, "Delay Time (s)"=w419) -> ("error out"=w420:errorcluster)  [unwired: 9 in]
            n157 = String Subset(string=w404, offset (0)=0, length (rest)=1 ("length (rest)")) -> (substring=w401:string)
            n158 = In Range and Coerce(upper limit=w431, x=w422, lower limit=w433) -> (In Range?=w430:bool)  [unwired: 1 out]
            n159 = To Double Precision Float(number=w422) -> (double precision float=w423:dbl)
            n160 = Not Equal?(x=w401, y="R") -> (x != y?=w400:bool)
            n161 = Equal?(x=w401, y="R") -> (x = y?=w418:bool)
            n162 = property on="Z in Motion" class="Bool (strict)"("Val(Sgnl)"=w400) -> ()  [unwired: 2 in, 2 out]
            n163 = property on="Z in Range" class="Bool (strict)"("Val(Sgnl)"=w430) -> ()  [unwired: 2 in, 2 out]
            n164 = property on="Z Ready" class="Bool (strict)"("Val(Sgnl)"=w418) -> ()  [unwired: 2 in, 2 out]
            n165 = Divide(x=w423, y=w429) -> (x/y=w427:dbl)
            n166 = property on="Z mm/rev" class="DigNum (strict)"() -> ("Value"=w426:dbl)  [unwired: 2 in, 2 out]
            n167 = Multiply(x=w427, y=w426) -> (x*y=w425:dbl)
            n168 = Add(x=w425, y=w424) -> (x+y=w421:dbl)
            n169 = property on="Z Position mm PV" class="DigNum (strict)"("Val(Sgnl)"=w421) -> ()  [unwired: 2 in, 2 out]
          }
          frame #1 {
            n170 = property on="Z Scan" class="Bool (strict)"() -> ("Value"=w436:bool)  [unwired: 2 in, 2 out]
            n171 = Or(x=w435, y=w436) -> (x .or. y?=w437:bool)
            n172 = case shown="True" w437 {
              frame False {
                n173 = property on="Z Scan OK" class="Bool"("DisabledEnum"=T2."Enabled" ("Disabled")) -> ()  [unwired: 2 in, 2 out]
                n174 = property on="Z Go" class="Bool"("DisabledEnum"=T2."Enabled" ("Disabled")) -> ()  [unwired: 2 in, 2 out]
              }
              frame True {
                n175 = property on="Z Scan OK" class="Bool"("DisabledEnum"=T2."Disabled and Grayed Out" ("Disabled")) -> ()  [unwired: 2 in, 2 out]
                n176 = property on="Z Go" class="Bool"("DisabledEnum"=T2."Disabled and Grayed Out" ("Disabled")) -> ()  [unwired: 2 in, 2 out]
              }
            }
          }
          frame #2 {
            n177 = case shown="False" w446 {
              tunnel: w447 -> [w454 w457]
              tunnel: [w452 w457] -> w448
              tunnel: [w451 w456] -> w449
              tunnel: w450 -> [w453 w456]
              frame False {
                n178 = call "Applied Send Command.vi"("error in (no error)"=w453, "Command"=T1."Stop & Kill Buffer", "VISA resource name"=w454) -> ("error out"=w451:errorcluster, "VISA resource name out"=w452:refnum<visa-resource-name>)  [unwired: 4 in, 1 out]
              }
              frame True {
              }
            }
          }
          frame #3 {
            n179 = disable-structure shown="Disabled" {
              disable-tunnel: w462 -> [w468 _]
              disable-tunnel: w461 -> [w466 _]
              disable-tunnel: w460 -> [w465 _]
              disable-tunnel: [w464 _] -> w459
              disable-tunnel: [w463 _] -> w458
              frame Disabled {
                n180 = property on="Z Backlash corr" class="Bool (strict)"() -> ("Value"=w469:bool)  [unwired: 2 in, 2 out]
                n181 = Implies(1:w468, 2:w469) -> (0:w467:bool)
                n182 = case shown="False" w467 {
                  tunnel: w466 -> [w470 w502]
                  tunnel: w465 -> [w471 w503]
                  tunnel: [w472 w502] -> w464
                  tunnel: [w473 w503] -> w463
                  frame False {
                    w499 = 0.1 ("Delay Time (s)")
                    # "Backlash"
                    # "Backlash"
                    n183 = property on="Z Backlash" class="DigNum (strict)"() -> ("Value"=w477:i32)  [unwired: 2 in, 2 out]
                    n184 = property on="Z Backlash corr" class="Bool (strict)"("Val(Sgnl)"=FALSE ("Value (Signaling)")) -> ()  [unwired: 2 in, 2 out]
                    n185 = To Long Integer(number=w477) -> (32bit integer=w480:i32)
                    n186 = Number To Decimal String(number=w477) -> (decimal integer string=w485:string)  [unwired: 1 in]
                    n187 = Negate(x=w480) -> (-x=w479:i32)
                    n188 = property on="Z Backlash steps/sec" class="DigNum (strict)"() -> ("Value"=w476:i32)  [unwired: 2 in, 2 out]
                    n189 = Number To Decimal String(number=w479) -> (decimal integer string=w486:string)  [unwired: 1 in]
                    n190 = property on="Z steps/rev" class="DigNum (strict)"() -> ("Value"=w475:u32)  [unwired: 2 in, 2 out]
                    n191 = Divide(x=w476, y=w475) -> (x/y=w500:dbl)
                    n192 = Number To Fractional String(number=w500) -> (F-format string=w501:string)  [unwired: 3 in]
                    n193 = call "Applied Send Command.vi"("error in (no error)"=w470, "Extra"=w501, "Command"=T1."Velocity Setting", "VISA resource name"=w471) -> ("error out"=w497:errorcluster, "VISA resource name out"=w490:refnum<visa-resource-name>)  [unwired: 3 in, 1 out]
                    n194 = call "Time Delay47"("error in (no error)"=w497, "Delay Time (s)"=w499) -> ("error out"=w498:errorcluster)  [unwired: 9 in]
                    n195 = call "Applied Send Command.vi"("error in (no error)"=w498, "Extra"=w485, "Command"=T1."Distance or Position", "VISA resource name"=w490) -> ("error out"=w491:errorcluster, "VISA resource name out"=w484:refnum<visa-resource-name>)  [unwired: 3 in, 1 out]
                    n196 = call "Time Delay44"("error in (no error)"=w491, "Delay Time (s)"=w499) -> ("error out"=w492:errorcluster)  [unwired: 9 in]
                    n197 = call "Applied Send Command.vi"("error in (no error)"=w492, "Command"=T1."Feed to Length", "VISA resource name"=w484) -> ("error out"=w493:errorcluster, "VISA resource name out"=w487:refnum<visa-resource-name>)  [unwired: 4 in, 1 out]
                    n198 = call "Time Delay45"("error in (no error)"=w493, "Delay Time (s)"=w499) -> ("error out"=w494:errorcluster)  [unwired: 9 in]
                    n199 = call "Applied Send Command.vi"("error in (no error)"=w494, "Extra"=w486, "Command"=T1."Distance or Position", "VISA resource name"=w487) -> ("error out"=w495:errorcluster, "VISA resource name out"=w488:refnum<visa-resource-name>)  [unwired: 3 in, 1 out]
                    n200 = call "Time Delay46"("error in (no error)"=w495, "Delay Time (s)"=w499) -> ("error out"=w496:errorcluster)  [unwired: 9 in]
                    n201 = call "Applied Send Command.vi"("error in (no error)"=w496, "Command"=T1."Feed to Length", "VISA resource name"=w488) -> ("error out"=w472:errorcluster, "VISA resource name out"=w473:refnum<visa-resource-name>)  [unwired: 4 in, 1 out]
                  }
                  frame True {
                  }
                }
              }
              frame Enabled {
              }
            }
          }
        }
        n202 = property on="X Step PV" class="DigNum (strict)"() -> ("Value"=w337:i32)  [unwired: 2 in, 2 out]
        n203 = property on="Y Step PV" class="DigNum (strict)"() -> ("Value"=w336:i32)  [unwired: 2 in, 2 out]
        n204 = Subtract(x=w338, y=w339) -> (x-y=w340:dbl)
        n205 = Absolute Value(x=w337) -> (abs(x)=w334:i32)
        n206 = Absolute Value(x=w336) -> (abs(x)=w335:i32)
        n207 = Subtract(x=w343, y=w342) -> (x-y=w344:dbl)
        n208 = property on="Y Scan Length SP steps" class="DigNum (strict)"() -> ("Value"=w346:i32)  [unwired: 2 in, 2 out]
        n209 = property on="Z Scan Length SP steps" class="DigNum (strict)"() -> ("Value"=w347:i32)  [unwired: 2 in, 2 out]
        n210 = Multiply(x=w334, y=w335) -> (x*y=w329:i32)
        n211 = Divide(x=w344, y=2.0) -> (x/y=w332:dbl)
        n212 = Divide(x=w340, y=2.0) -> (x/y=w333:dbl)
        n213 = Absolute Value(x=w332) -> (abs(x)=w330:dbl)
        n214 = Absolute Value(x=w333) -> (abs(x)=w331:dbl)
        n215 = Divide(x=w346, y=w347) -> (x/y=w348:dbl)
        n216 = Multiply(x=w330, y=w331) -> (x*y=w328:dbl)
        n217 = Inverse Tangent(1:w348) -> (0:w349:dbl)
        n218 = Less Or Equal?(x=w329, y=w328) -> (x <= y?=w327:bool)
        n219 = Divide(x=w349, y=6.283185307179586) -> (x/y=w350:dbl)
        n220 = flat-sequence {
          tunnel: [w516] -> w384
          tunnel: [w527] -> w383
          tunnel: [w505] -> w382
          tunnel: [w512] -> w381
          tunnel: w354 -> [w523]
          tunnel: w373 -> [w511]
          tunnel: w338 -> [w507]
          tunnel: w339 -> [w506]
          tunnel: w327 -> [w504]
          tunnel: w384 -> [w547]
          tunnel: [w547] -> w380
          tunnel: w383 -> [w546]
          tunnel: [w546] -> w379
          tunnel: w382 -> [w545]
          tunnel: [w545] -> w378
          tunnel: w381 -> [w542]
          tunnel: [w542] -> w377
          tunnel: w380 -> [w556]
          tunnel: [w553] -> w376
          tunnel: w379 -> [w555]
          tunnel: [w554] -> w375
          tunnel: w378 -> [w552]
          tunnel: [w557] -> w374
          tunnel: w377 -> [w557]
          tunnel: w376 -> [w567]
          tunnel: w375 -> [w568]
          tunnel: w374 -> [w569]
          tunnel: [w566] -> w371
          tunnel: [w565] -> w372
          frame #0 {
            w526 = 0.2 ("Delay Time (s)")
            n221 = To Long Integer(number=w507) -> (32bit integer=w539:i32)
            n222 = To Long Integer(number=w506) -> (32bit integer=w540:i32)
            n223 = property on="X steps/rev" class="DigNum (strict)"() -> ("Value"=w536:u32)  [unwired: 2 in, 2 out]
            n224 = property on="X offset mm" class="DigNum (strict)"() -> ("Value"=w532:dbl)  [unwired: 2 in, 2 out]
            n225 = To Double Precision Float(number=w536) -> (double precision float=w537:dbl)
            n226 = call "Applied Send Command.vi"("error in (no error)"=w511, "Command"=T1."Immediate Position?", "VISA resource name"=w523) -> ("error out"=w521:errorcluster, "read buffer"=w522:string, "VISA resource name out"=w517:refnum<visa-resource-name>)  [unwired: 4 in]
            n227 = call "Time Delay12"("error in (no error)"=w521, "Delay Time (s)"=w526) -> ("error out"=w514:errorcluster)  [unwired: 9 in]
            n228 = Hexadecimal String To Number(string=w522, offset=3) -> (number=w528:u32)  [unwired: 1 in, 1 out]
            n229 = To Long Integer(number=w528) -> (32bit integer=w530:i32)
            n230 = call "Applied Send Command.vi"("error in (no error)"=w514, "Command"=T1."Request Status", "VISA resource name"=w517) -> ("error out"=w515:errorcluster, "read buffer"=w519:string, "VISA resource name out"=w516:refnum<visa-resource-name>)  [unwired: 4 in]
            n231 = property on="X Step PV" class="DigNum (strict)"("Val(Sgnl)"=w530) -> ()  [unwired: 2 in, 2 out]
            n232 = call "Time Delay11"("error in (no error)"=w515, "Delay Time (s)"=w526) -> ("error out"=w527:errorcluster)  [unwired: 9 in]
            n233 = String Subset(string=w519, offset (0)=0, length (rest)=1 ("length (rest)")) -> (substring=w508:string)
            n234 = In Range and Coerce(upper limit=w539, x=w530, lower limit=w540) -> (In Range?=w538:bool)  [unwired: 1 out]
            n235 = To Double Precision Float(number=w530) -> (double precision float=w531:dbl)
            n236 = Not Equal?(x=w508, y="R") -> (x != y?=w512:bool)
            n237 = Equal?(x=w508, y="R") -> (x = y?=w525:bool)
            n238 = property on="X  in Motion" class="Bool (strict)"("Val(Sgnl)"=w512) -> ()  [unwired: 2 in, 2 out]
            n239 = property on="X Ready" class="Bool (strict)"("Val(Sgnl)"=w525) -> ()  [unwired: 2 in, 2 out]
            n240 = Divide(x=w531, y=w537) -> (x/y=w535:dbl)
            n241 = And(x=w504, y=w538) -> (x .and. y?=w505:bool)
            n242 = property on="X  in Range" class="Bool (strict)"("Val(Sgnl)"=w505) -> ()  [unwired: 2 in, 2 out]
            n243 = property on="X mm/rev" class="DigNum (strict)"() -> ("Value"=w534:dbl)  [unwired: 2 in, 2 out]
            n244 = Multiply(x=w535, y=w534) -> (x*y=w533:dbl)
            n245 = Add(x=w533, y=w532) -> (x+y=w529:dbl)
            n246 = property on="X Position mm PV" class="DigNum (strict)"("Val(Sgnl)"=w529) -> ()  [unwired: 2 in, 2 out]
          }
          frame #1 {
            n247 = property on="X Scan" class="Bool (strict)"() -> ("Value"=w543:bool)  [unwired: 2 in, 2 out]
            n248 = Or(x=w542, y=w543) -> (x .or. y?=w544:bool)
            n249 = case shown="True" w544 {
              frame False {
                n250 = property on="X Scan OK" class="Bool"("DisabledEnum"=T2."Enabled" ("Disabled")) -> ()  [unwired: 2 in, 2 out]
                n251 = property on="X Go" class="Bool"("DisabledEnum"=T2."Enabled" ("Disabled")) -> ()  [unwired: 2 in, 2 out]
              }
              frame True {
                n252 = property on="X Scan OK" class="Bool"("DisabledEnum"=T2."Disabled and Grayed Out" ("Disabled")) -> ()  [unwired: 2 in, 2 out]
                n253 = property on="X Go" class="Bool"("DisabledEnum"=T2."Disabled and Grayed Out" ("Disabled")) -> ()  [unwired: 2 in, 2 out]
              }
            }
          }
          frame #2 {
            n254 = case shown="False" w552 {
              tunnel: w556 -> [w559 w564]
              tunnel: [w561 w564] -> w553
              tunnel: [w562 w563] -> w554
              tunnel: w555 -> [w558 w563]
              frame False {
                n255 = call "Applied Send Command.vi"("error in (no error)"=w558, "Command"=T1."Stop & Kill Buffer", "VISA resource name"=w559) -> ("error out"=w562:errorcluster, "VISA resource name out"=w561:refnum<visa-resource-name>)  [unwired: 4 in, 1 out]
              }
              frame True {
              }
            }
          }
          frame #3 {
            n256 = disable-structure shown="Disabled" {
              disable-tunnel: w569 -> [w575 _]
              disable-tunnel: w568 -> [w574 _]
              disable-tunnel: w567 -> [w573 _]
              disable-tunnel: [w572 _] -> w566
              disable-tunnel: [w571 _] -> w565
              frame Disabled {
                n257 = property on="X Backlash corr" class="Bool (strict)"() -> ("Value"=w576:bool)  [unwired: 2 in, 2 out]
                n258 = Implies(1:w575, 2:w576) -> (0:w570:bool)
                n259 = case shown="False" w570 {
                  tunnel: w574 -> [w590 w609]
                  tunnel: w573 -> [w591 w610]
                  tunnel: [w593 w609] -> w572
                  tunnel: [w592 w610] -> w571
                  frame False {
                    w581 = 0.1 ("Delay Time (s)")
                    # "Backlash"
                    n260 = property on="X Backlash" class="DigNum (strict)"() -> ("Value"=w596:i32)  [unwired: 2 in, 2 out]
                    n261 = property on="X Backlash corr" class="Bool (strict)"("Val(Sgnl)"=FALSE ("Value (Signaling)")) -> ()  [unwired: 2 in, 2 out]
                    n262 = To Long Integer(number=w596) -> (32bit integer=w605:i32)
                    n263 = Number To Decimal String(number=w596) -> (decimal integer string=w600:string)  [unwired: 1 in]
                    n264 = Negate(x=w605) -> (-x=w606:i32)
                    n265 = property on="X Backlash steps/sec" class="DigNum (strict)"() -> ("Value"=w580:i32)  [unwired: 2 in, 2 out]
                    n266 = Number To Decimal String(number=w606) -> (decimal integer string=w599:string)  [unwired: 1 in]
                    n267 = property on="X steps/rev" class="DigNum (strict)"() -> ("Value"=w579:u32)  [unwired: 2 in, 2 out]
                    n268 = Divide(x=w580, y=w579) -> (x/y=w578:dbl)
                    n269 = Number To Fractional String(number=w578) -> (F-format string=w577:string)  [unwired: 3 in]
                    n270 = call "Applied Send Command.vi"("error in (no error)"=w590, "Extra"=w577, "Command"=T1."Velocity Setting", "VISA resource name"=w591) -> ("error out"=w583:errorcluster, "VISA resource name out"=w594:refnum<visa-resource-name>)  [unwired: 3 in, 1 out]
                    n271 = call "Time Delay35"("error in (no error)"=w583, "Delay Time (s)"=w581) -> ("error out"=w582:errorcluster)  [unwired: 9 in]
                    n272 = call "Applied Send Command.vi"("error in (no error)"=w582, "Extra"=w600, "Command"=T1."Distance or Position", "VISA resource name"=w594) -> ("error out"=w589:errorcluster, "VISA resource name out"=w601:refnum<visa-resource-name>)  [unwired: 3 in, 1 out]
                    n273 = call "Time Delay32"("error in (no error)"=w589, "Delay Time (s)"=w581) -> ("error out"=w588:errorcluster)  [unwired: 9 in]
                    n274 = call "Applied Send Command.vi"("error in (no error)"=w588, "Command"=T1."Feed to Length", "VISA resource name"=w601) -> ("error out"=w587:errorcluster, "VISA resource name out"=w598:refnum<visa-resource-name>)  [unwired: 4 in, 1 out]
                    n275 = call "Time Delay33"("error in (no error)"=w587, "Delay Time (s)"=w581) -> ("error out"=w586:errorcluster)  [unwired: 9 in]
                    n276 = call "Applied Send Command.vi"("error in (no error)"=w586, "Extra"=w599, "Command"=T1."Distance or Position", "VISA resource name"=w598) -> ("error out"=w585:errorcluster, "VISA resource name out"=w597:refnum<visa-resource-name>)  [unwired: 3 in, 1 out]
                    n277 = call "Time Delay34"("error in (no error)"=w585, "Delay Time (s)"=w581) -> ("error out"=w584:errorcluster)  [unwired: 9 in]
                    n278 = call "Applied Send Command.vi"("error in (no error)"=w584, "Command"=T1."Feed to Length", "VISA resource name"=w597) -> ("error out"=w593:errorcluster, "VISA resource name out"=w592:refnum<visa-resource-name>)  [unwired: 4 in, 1 out]
                  }
                  frame True {
                  }
                }
              }
              frame Enabled {
              }
            }
          }
        }
        n279 = flat-sequence {
          tunnel: w398 -> [w627]
          tunnel: w355 -> [w628]
          tunnel: [w624] -> w395
          tunnel: [w634] -> w393
          tunnel: [w613] -> w391
          tunnel: [w615] -> w389
          tunnel: w343 -> [w614]
          tunnel: w342 -> [w611]
          tunnel: w327 -> [w612]
          tunnel: w395 -> [w654]
          tunnel: [w654] -> w394
          tunnel: w393 -> [w653]
          tunnel: [w653] -> w392
          tunnel: w391 -> [w652]
          tunnel: [w652] -> w390
          tunnel: w389 -> [w649]
          tunnel: [w649] -> w385
          tunnel: w394 -> [w661]
          tunnel: [w662] -> w388
          tunnel: w392 -> [w664]
          tunnel: [w663] -> w387
          tunnel: w390 -> [w660]
          tunnel: [w659] -> w386
          tunnel: w385 -> [w659]
          tunnel: w388 -> [w674]
          tunnel: w387 -> [w675]
          tunnel: w386 -> [w676]
          tunnel: [w673] -> w397
          tunnel: [w672] -> w396
          frame #0 {
            w633 = 0.2 ("Delay Time (s)")
            n280 = To Long Integer(number=w614) -> (32bit integer=w646:i32)
            n281 = To Long Integer(number=w611) -> (32bit integer=w647:i32)
            n282 = property on="Y steps/rev" class="DigNum (strict)"() -> ("Value"=w643:u32)  [unwired: 2 in, 2 out]
            n283 = property on="Y offset mm" class="DigNum (strict)"() -> ("Value"=w639:dbl)  [unwired: 2 in, 2 out]
            n284 = To Double Precision Float(number=w643) -> (double precision float=w644:dbl)
            n285 = call "Applied Send Command.vi"("error in (no error)"=w627, "Command"=T1."Immediate Position?", "VISA resource name"=w628) -> ("error out"=w630:errorcluster, "read buffer"=w631:string, "VISA resource name out"=w625:refnum<visa-resource-name>)  [unwired: 4 in]
            n286 = call "Time Delay4"("error in (no error)"=w630, "Delay Time (s)"=w633) -> ("error out"=w623:errorcluster)  [unwired: 9 in]
            n287 = Hexadecimal String To Number(string=w631, offset=3) -> (number=w635:u32)  [unwired: 1 in, 1 out]
            n288 = To Long Integer(number=w635) -> (32bit integer=w637:i32)
            n289 = call "Applied Send Command.vi"("error in (no error)"=w623, "Command"=T1."Request Status", "VISA resource name"=w625) -> ("error out"=w622:errorcluster, "read buffer"=w619:string, "VISA resource name out"=w624:refnum<visa-resource-name>)  [unwired: 4 in]
            n290 = property on="Y Step PV" class="DigNum (strict)"("Val(Sgnl)"=w637) -> ()  [unwired: 2 in, 2 out]
            n291 = call "Time Delay3"("error in (no error)"=w622, "Delay Time (s)"=w633) -> ("error out"=w634:errorcluster)  [unwired: 9 in]
            n292 = String Subset(string=w619, offset (0)=0, length (rest)=1 ("length (rest)")) -> (substring=w617:string)
            n293 = In Range and Coerce(upper limit=w646, x=w637, lower limit=w647) -> (In Range?=w645:bool)  [unwired: 1 out]
            n294 = To Double Precision Float(number=w637) -> (double precision float=w638:dbl)
            n295 = Not Equal?(x=w617, y="R") -> (x != y?=w615:bool)
            n296 = Equal?(x=w617, y="R") -> (x = y?=w632:bool)
            n297 = property on="Y in Motion" class="Bool (strict)"("Val(Sgnl)"=w615) -> ()  [unwired: 2 in, 2 out]
            n298 = property on="Y Ready" class="Bool (strict)"("Val(Sgnl)"=w632) -> ()  [unwired: 2 in, 2 out]
            n299 = Divide(x=w638, y=w644) -> (x/y=w642:dbl)
            n300 = And(x=w645, y=w612) -> (x .and. y?=w613:bool)
            n301 = property on="Y in Range" class="Bool (strict)"("Val(Sgnl)"=w613) -> ()  [unwired: 2 in, 2 out]
            n302 = property on="Y mm/rev" class="DigNum (strict)"() -> ("Value"=w641:dbl)  [unwired: 2 in, 2 out]
            n303 = Multiply(x=w642, y=w641) -> (x*y=w640:dbl)
            n304 = Add(x=w640, y=w639) -> (x+y=w636:dbl)
            n305 = property on="Y Position mm PV" class="DigNum (strict)"("Val(Sgnl)"=w636) -> ()  [unwired: 2 in, 2 out]
          }
          frame #1 {
            n306 = property on="Y Scan" class="Bool (strict)"() -> ("Value"=w650:bool)  [unwired: 2 in, 2 out]
            n307 = Or(x=w649, y=w650) -> (x .or. y?=w651:bool)
            n308 = case shown="True" w651 {
              frame False {
                n309 = property on="Y Scan OK" class="Bool"("DisabledEnum"=T2."Enabled" ("Disabled")) -> ()  [unwired: 2 in, 2 out]
                n310 = property on="Y Go" class="Bool"("DisabledEnum"=T2."Enabled" ("Disabled")) -> ()  [unwired: 2 in, 2 out]
              }
              frame True {
                n311 = property on="Y Scan OK" class="Bool"("DisabledEnum"=T2."Disabled and Grayed Out" ("Disabled")) -> ()  [unwired: 2 in, 2 out]
                n312 = property on="Y Go" class="Bool"("DisabledEnum"=T2."Disabled and Grayed Out" ("Disabled")) -> ()  [unwired: 2 in, 2 out]
              }
            }
          }
          frame #2 {
            n313 = case shown="False" w660 {
              tunnel: w661 -> [w666 w671]
              tunnel: [w668 w671] -> w662
              tunnel: [w667 w670] -> w663
              tunnel: w664 -> [w665 w670]
              frame False {
                n314 = call "Applied Send Command.vi"("error in (no error)"=w665, "Command"=T1."Stop & Kill Buffer", "VISA resource name"=w666) -> ("error out"=w667:errorcluster, "VISA resource name out"=w668:refnum<visa-resource-name>)  [unwired: 4 in, 1 out]
              }
              frame True {
              }
            }
          }
          frame #3 {
            n315 = disable-structure shown="Disabled" {
              disable-tunnel: w676 -> [w682 _]
              disable-tunnel: w675 -> [w680 _]
              disable-tunnel: w674 -> [w679 _]
              disable-tunnel: [w678 _] -> w673
              disable-tunnel: [w677 _] -> w672
              frame Disabled {
                n316 = property on="Y Backlash corr" class="Bool (strict)"() -> ("Value"=w683:bool)  [unwired: 2 in, 2 out]
                n317 = Implies(1:w682, 2:w683) -> (0:w681:bool)
                n318 = case shown="False" w681 {
                  tunnel: w680 -> [w686 w715]
                  tunnel: w679 -> [w687 w716]
                  tunnel: [w684 w715] -> w678
                  tunnel: [w685 w716] -> w677
                  frame False {
                    w693 = 0.1 ("Delay Time (s)")
                    # "Backlash"
                    n319 = property on="Y Backlash" class="DigNum (strict)"() -> ("Value"=w688:i32)  [unwired: 2 in, 2 out]
                    n320 = property on="Y Backlash corr" class="Bool (strict)"("Val(Sgnl)"=FALSE ("Value (Signaling)")) -> ()  [unwired: 2 in, 2 out]
                    n321 = To Long Integer(number=w688) -> (32bit integer=w711:i32)
                    n322 = Number To Decimal String(number=w688) -> (decimal integer string=w706:string)  [unwired: 1 in]
                    n323 = Negate(x=w711) -> (-x=w712:i32)
                    n324 = property on="Y Backlash steps/sec" class="DigNum (strict)"() -> ("Value"=w689:i32)  [unwired: 2 in, 2 out]
                    n325 = Number To Decimal String(number=w712) -> (decimal integer string=w705:string)  [unwired: 1 in]
                    n326 = property on="Y steps/rev" class="DigNum (strict)"() -> ("Value"=w692:u32)  [unwired: 2 in, 2 out]
                    n327 = Divide(x=w689, y=w692) -> (x/y=w691:dbl)
                    n328 = Number To Fractional String(number=w691) -> (F-format string=w690:string)  [unwired: 3 in]
                    n329 = call "Applied Send Command.vi"("error in (no error)"=w686, "Extra"=w690, "Command"=T1."Velocity Setting", "VISA resource name"=w687) -> ("error out"=w695:errorcluster, "VISA resource name out"=w701:refnum<visa-resource-name>)  [unwired: 3 in, 1 out]
                    n330 = call "Time Delay41"("error in (no error)"=w695, "Delay Time (s)"=w693) -> ("error out"=w694:errorcluster)  [unwired: 9 in]
                    n331 = call "Applied Send Command.vi"("error in (no error)"=w694, "Extra"=w706, "Command"=T1."Distance or Position", "VISA resource name"=w701) -> ("error out"=w700:errorcluster, "VISA resource name out"=w707:refnum<visa-resource-name>)  [unwired: 3 in, 1 out]
                    n332 = call "Time Delay38"("error in (no error)"=w700, "Delay Time (s)"=w693) -> ("error out"=w699:errorcluster)  [unwired: 9 in]
                    n333 = call "Applied Send Command.vi"("error in (no error)"=w699, "Command"=T1."Feed to Length", "VISA resource name"=w707) -> ("error out"=w698:errorcluster, "VISA resource name out"=w704:refnum<visa-resource-name>)  [unwired: 4 in, 1 out]
                    n334 = call "Applied Send Command.vi"("Extra"=w705, "Command"=T1."Distance or Position", "VISA resource name"=w704) -> ("error out"=w697:errorcluster, "VISA resource name out"=w703:refnum<visa-resource-name>)  [unwired: 4 in, 1 out]
                    n335 = call "Time Delay39"("error in (no error)"=w698, "Delay Time (s)"=w693) -> ()  [unwired: 9 in, 1 out]
                    n336 = call "Time Delay40"("error in (no error)"=w697, "Delay Time (s)"=w693) -> ("error out"=w696:errorcluster)  [unwired: 9 in]
                    n337 = call "Applied Send Command.vi"("error in (no error)"=w696, "Command"=T1."Feed to Length", "VISA resource name"=w703) -> ("error out"=w684:errorcluster, "VISA resource name out"=w685:refnum<visa-resource-name>)  [unwired: 4 in, 1 out]
                  }
                  frame True {
                  }
                }
              }
              frame Enabled {
              }
            }
          }
        }
        n338 = Multiply(x=360.0, y=w350) -> (x*y=w353:dbl)
        n339 = property on="atan Y/Z" class="DigNum (strict)"("Val(Sgnl)"=w353) -> ()  [unwired: 2 in, 2 out]
      }
      event "Reset Y Position mm", "Reset X Position mm", "Reset Z Position mm": Value Change {
        n340 = event-data() -> ()  [unwired: 1 in, 5 out]
        n341 = property on="Z steps/rev" class="DigNum (strict)"() -> ("Value"=w719:u32)  [unwired: 2 in, 2 out]
        n342 = property on="X steps/rev" class="DigNum (strict)"() -> ("Value"=w728:u32)  [unwired: 2 in, 2 out]
        n343 = property on="Y steps/rev" class="DigNum (strict)"() -> ("Value"=w737:u32)  [unwired: 2 in, 2 out]
        n344 = property on="Z offset mm" class="DigNum (strict)"() -> ("Value"=w717:dbl)  [unwired: 2 in, 2 out]
        n345 = property on="X offset mm" class="DigNum (strict)"() -> ("Value"=w726:dbl)  [unwired: 2 in, 2 out]
        n346 = property on="Y offset mm" class="DigNum (strict)"() -> ("Value"=w735:dbl)  [unwired: 2 in, 2 out]
        n347 = To Double Precision Float(number=w728) -> (double precision float=w731:dbl)
        n348 = To Double Precision Float(number=w737) -> (double precision float=w740:dbl)
        n349 = property on="Reset Z Position mm" class="DigNum (strict)"() -> ("Value"=w725:dbl)  [unwired: 2 in, 2 out]
        n350 = property on="Reset X Position mm" class="DigNum (strict)"() -> ("Value"=w734:dbl)  [unwired: 2 in, 2 out]
        n351 = property on="Reset Y Position mm" class="DigNum (strict)"() -> ("Value"=w743:dbl)  [unwired: 2 in, 2 out]
        n352 = Subtract(x=w725, y=w717) -> (x-y=w724:dbl)
        n353 = Subtract(x=w734, y=w726) -> (x-y=w733:dbl)
        n354 = Subtract(x=w743, y=w735) -> (x-y=w742:dbl)
        n355 = property on="Z mm/rev" class="DigNum (strict)"() -> ("Value"=w718:dbl)  [unwired: 2 in, 2 out]
        n356 = property on="X mm/rev" class="DigNum (strict)"() -> ("Value"=w727:dbl)  [unwired: 2 in, 2 out]
        n357 = property on="Y mm/rev" class="DigNum (strict)"() -> ("Value"=w736:dbl)  [unwired: 2 in, 2 out]
        n358 = Divide(x=w733, y=w727) -> (x/y=w732:dbl)
        n359 = Divide(x=w742, y=w736) -> (x/y=w741:dbl)
        n360 = Divide(x=w724, y=w718) -> (x/y=w723:dbl)
        n361 = To Double Precision Float(number=w719) -> (double precision float=w722:dbl)
        n362 = Multiply(x=w723, y=w722) -> (x*y=w721:dbl)
        n363 = Multiply(x=w732, y=w731) -> (x*y=w730:dbl)
        n364 = Multiply(x=w741, y=w740) -> (x*y=w739:dbl)
        n365 = To Long Integer(number=w721) -> (32bit integer=w720:i32)
        n366 = To Long Integer(number=w730) -> (32bit integer=w729:i32)
        n367 = To Long Integer(number=w739) -> (32bit integer=w738:i32)
        n368 = property on="Reset Z Motor Steps" class="DigNum (strict)"("Val(Sgnl)"=w720) -> ()  [unwired: 2 in, 2 out]
        n369 = property on="Reset X Motor Steps" class="DigNum (strict)"("Val(Sgnl)"=w729) -> ()  [unwired: 2 in, 2 out]
        n370 = property on="Reset Y Motor Steps" class="DigNum (strict)"("Val(Sgnl)"=w738) -> ()  [unwired: 2 in, 2 out]
      }
      event "Y Velocity SP step/sec", "X Velocity SP step/sec", "Z Velocity SP step/sec", "Y Step SP", "X Step SP", "Z Step SP": Value Change {
        n371 = event-data() -> ()  [unwired: 1 in, 5 out]
        n372 = property on="Z Step SP" class="DigNum (strict)"() -> ("Value"=w750:i32)  [unwired: 2 in, 2 out]
        n373 = property on="Y Step SP" class="DigNum (strict)"() -> ("Value"=w766:i32)  [unwired: 2 in, 2 out]
        n374 = property on="X Step SP" class="DigNum (strict)"() -> ("Value"=w758:i32)  [unwired: 2 in, 2 out]
        n375 = property on="Z steps/rev" class="DigNum (strict)"() -> ("Value"=w771:u32)  [unwired: 2 in, 2 out]
        n376 = property on="Z steps/rev" class="DigNum (strict)"() -> ("Value"=w748:u32)  [unwired: 2 in, 2 out]
        n377 = property on="Y steps/rev" class="DigNum (strict)"() -> ("Value"=w783:u32)  [unwired: 2 in, 2 out]
        n378 = property on="Y steps/rev" class="DigNum (strict)"() -> ("Value"=w764:u32)  [unwired: 2 in, 2 out]
        n379 = property on="X steps/rev" class="DigNum (strict)"() -> ("Value"=w777:u32)  [unwired: 2 in, 2 out]
        n380 = property on="X steps/rev" class="DigNum (strict)"() -> ("Value"=w756:u32)  [unwired: 2 in, 2 out]
        n381 = property on="Z offset mm" class="DigNum (strict)"() -> ("Value"=w747:dbl)  [unwired: 2 in, 2 out]
        n382 = property on="Y offset mm" class="DigNum (strict)"() -> ("Value"=w763:dbl)  [unwired: 2 in, 2 out]
        n383 = property on="X offset mm" class="DigNum (strict)"() -> ("Value"=w755:dbl)  [unwired: 2 in, 2 out]
        n384 = To Double Precision Float(number=w771) -> (double precision float=w776:dbl)
        n385 = To Double Precision Float(number=w750) -> (double precision float=w751:dbl)
        n386 = To Double Precision Float(number=w748) -> (double precision float=w754:dbl)
        n387 = To Double Precision Float(number=w766) -> (double precision float=w767:dbl)
        n388 = To Double Precision Float(number=w764) -> (double precision float=w770:dbl)
        n389 = To Double Precision Float(number=w777) -> (double precision float=w782:dbl)
        n390 = To Double Precision Float(number=w758) -> (double precision float=w759:dbl)
        n391 = To Double Precision Float(number=w756) -> (double precision float=w762:dbl)
        n392 = Divide(x=w751, y=w754) -> (x/y=w753:dbl)
        n393 = Divide(x=w767, y=w770) -> (x/y=w769:dbl)
        n394 = Divide(x=w759, y=w762) -> (x/y=w761:dbl)
        n395 = property on="Z Velocity SP step/sec" class="DigNum (strict)"() -> ("Value"=w773:i32)  [unwired: 2 in, 2 out]
        n396 = property on="Z mm/rev" class="DigNum (strict)"() -> ("Value"=w746:dbl)  [unwired: 2 in, 2 out]
        n397 = property on="Y Velocity SP step/sec" class="DigNum (strict)"() -> ("Value"=w785:i32)  [unwired: 2 in, 2 out]
        n398 = property on="Y mm/rev" class="DigNum (strict)"() -> ("Value"=w744:dbl)  [unwired: 2 in, 2 out]
        n399 = property on="X Velocity SP step/sec" class="DigNum (strict)"() -> ("Value"=w779:i32)  [unwired: 2 in, 2 out]
        n400 = property on="X mm/rev" class="DigNum (strict)"() -> ("Value"=w745:dbl)  [unwired: 2 in, 2 out]
        n401 = Multiply(x=w753, y=w746) -> (x*y=w752:dbl)
        n402 = Multiply(x=w769, y=w744) -> (x*y=w768:dbl)
        n403 = Multiply(x=w761, y=w745) -> (x*y=w760:dbl)
        n404 = To Double Precision Float(number=w773) -> (double precision float=w774:dbl)
        n405 = To Double Precision Float(number=w785) -> (double precision float=w786:dbl)
        n406 = To Double Precision Float(number=w783) -> (double precision float=w788:dbl)
        n407 = To Double Precision Float(number=w779) -> (double precision float=w780:dbl)
        n408 = Divide(x=w774, y=w776) -> (x/y=w775:dbl)
        n409 = Add(x=w752, y=w747) -> (x+y=w749:dbl)
        n410 = Divide(x=w786, y=w788) -> (x/y=w787:dbl)
        n411 = Add(x=w768, y=w763) -> (x+y=w765:dbl)
        n412 = Divide(x=w780, y=w782) -> (x/y=w781:dbl)
        n413 = Add(x=w760, y=w755) -> (x+y=w757:dbl)
        n414 = Multiply(x=w775, y=w746) -> (x*y=w772:dbl)
        n415 = property on="Z Position MV mm" class="DigNum (strict)"("Val(Sgnl)"=w749) -> ()  [unwired: 2 in, 2 out]
        n416 = Multiply(x=w787, y=w744) -> (x*y=w784:dbl)
        n417 = property on="Y Position MV mm" class="DigNum (strict)"("Val(Sgnl)"=w765) -> ()  [unwired: 2 in, 2 out]
        n418 = Multiply(x=w781, y=w745) -> (x*y=w778:dbl)
        n419 = property on="X Position MV mm" class="DigNum (strict)"("Val(Sgnl)"=w757) -> ()  [unwired: 2 in, 2 out]
        n420 = property on="Z Velocity MV mm/sec" class="DigNum (strict)"("Val(Sgnl)"=w772) -> ()  [unwired: 2 in, 2 out]
        n421 = property on="Y Velocity MV mm/sec" class="DigNum (strict)"("Val(Sgnl)"=w784) -> ()  [unwired: 2 in, 2 out]
        n422 = property on="X Velocity MV mm/sec" class="DigNum (strict)"("Val(Sgnl)"=w778) -> ()  [unwired: 2 in, 2 out]
      }
      event "Y Scan Length SP steps", "Y Scan Velocity SP steps/sec", "X Scan Velocity SP steps/sec", "X Scan Length SP steps", "Z Scan Velocity SP steps/sec", "Z Scan Length SP steps": Value Change {
        n423 = event-data() -> ()  [unwired: 1 in, 5 out]
        n424 = property on="Z steps/rev" class="DigNum (strict)"() -> ("Value"=w812:u32)  [unwired: 2 in, 2 out]
        n425 = property on="X steps/rev" class="DigNum (strict)"() -> ("Value"=w839:u32)  [unwired: 2 in, 2 out]
        n426 = property on="Y steps/rev" class="DigNum (strict)"() -> ("Value"=w825:u32)  [unwired: 2 in, 2 out]
        n427 = property on="X Step PV" class="DigNum (strict)"() -> ("Value"=w837:i32)  [unwired: 2 in, 2 out]
        n428 = property on="Y Step PV" class="DigNum (strict)"() -> ("Value"=w823:i32)  [unwired: 2 in, 2 out]
        n429 = property on="Z Step PV" class="DigNum (strict)"() -> ("Value"=w810:i32)  [unwired: 2 in, 2 out]
        n430 = To Double Precision Float(number=w837) -> (double precision float=w804:dbl)
        n431 = To Double Precision Float(number=w823) -> (double precision float=w803:dbl)
        n432 = To Double Precision Float(number=w810) -> (double precision float=w802:dbl)
        n433 = To Double Precision Float(number=w812) -> (double precision float=w809:dbl)
        n434 = To Double Precision Float(number=w839) -> (double precision float=w836:dbl)
        n435 = To Double Precision Float(number=w825) -> (double precision float=w798:dbl)
        n436 = property on="X Step SP" class="DigNum (strict)"() -> ("Maximum"=w843:dbl)  [unwired: 2 in, 2 out]
        n437 = property on="Y Step SP" class="DigNum (strict)"() -> ("Maximum"=w829:dbl)  [unwired: 2 in, 2 out]
        n438 = property on="Z Step SP" class="DigNum (strict)"() -> ("Maximum"=w816:dbl)  [unwired: 2 in, 2 out]
        n439 = property on="X Step SP" class="DigNum (strict)"() -> ("Minimum"=w844:dbl)  [unwired: 2 in, 2 out]
        n440 = property on="Y Step SP" class="DigNum (strict)"() -> ("Minimum"=w830:dbl)  [unwired: 2 in, 2 out]
        n441 = property on="Z Step SP" class="DigNum (strict)"() -> ("Minimum"=w817:dbl)  [unwired: 2 in, 2 out]
        n442 = property on="Z Scan Length SP steps" class="DigNum (strict)"() -> ("Value"=w813:i32)  [unwired: 2 in, 2 out]
        n443 = property on="X Scan Length SP steps" class="DigNum (strict)"() -> ("Value"=w835:i32)  [unwired: 2 in, 2 out]
        n444 = property on="Y Scan Length SP steps" class="DigNum (strict)"() -> ("Value"=w826:i32)  [unwired: 2 in, 2 out]
        n445 = property on="Z Scan Velocity SP steps/sec" class="DigNum (strict)"() -> ("Value"=w808:i32)  [unwired: 2 in, 2 out]
        n446 = property on="X Scan Velocity SP steps/sec" class="DigNum (strict)"() -> ("Value"=w840:i32)  [unwired: 2 in, 2 out]
        n447 = property on="Y Scan Velocity SP steps/sec" class="DigNum (strict)"() -> ("Value"=w822:i32)  [unwired: 2 in, 2 out]
        n448 = Subtract(x=w844, y=w804) -> (x-y=w845:dbl)
        n449 = Subtract(x=w843, y=w804) -> (x-y=w842:dbl)
        n450 = Subtract(x=w830, y=w803) -> (x-y=w831:dbl)
        n451 = Subtract(x=w829, y=w803) -> (x-y=w828:dbl)
        n452 = Subtract(x=w817, y=w802) -> (x-y=w818:dbl)
        n453 = Subtract(x=w816, y=w802) -> (x-y=w815:dbl)
        n454 = To Double Precision Float(number=w813) -> (double precision float=w801:dbl)
        n455 = To Double Precision Float(number=w835) -> (double precision float=w793:dbl)
        n456 = To Double Precision Float(number=w826) -> (double precision float=w797:dbl)
        n457 = property on="X Scan Length SP steps" class="DigNum (strict)"("Minimum"=w845) -> ()  [unwired: 2 in, 2 out]
        n458 = property on="Y Scan Length SP steps" class="DigNum (strict)"("Minimum"=w831) -> ()  [unwired: 2 in, 2 out]
        n459 = property on="Z Scan Length SP steps" class="DigNum (strict)"("Minimum"=w818) -> ()  [unwired: 2 in, 2 out]
        n460 = property on="X Scan Length SP steps" class="DigNum (strict)"("Maximum"=w842) -> ()  [unwired: 2 in, 2 out]
        n461 = property on="Y Scan Length SP steps" class="DigNum (strict)"("Maximum"=w828) -> ()  [unwired: 2 in, 2 out]
        n462 = property on="Z Scan Length SP steps" class="DigNum (strict)"("Maximum"=w815) -> ()  [unwired: 2 in, 2 out]
        n463 = Divide(x=w801, y=w809) -> (x/y=w814:dbl)
        n464 = Divide(x=w793, y=w836) -> (x/y=w834:dbl)
        n465 = Divide(x=w797, y=w798) -> (x/y=w827:dbl)
        n466 = To Double Precision Float(number=w808) -> (double precision float=w800:dbl)
        n467 = To Double Precision Float(number=w840) -> (double precision float=w792:dbl)
        n468 = To Double Precision Float(number=w822) -> (double precision float=w796:dbl)
        n469 = property on="Z mm/rev" class="DigNum (strict)"() -> ("Value"=w811:dbl)  [unwired: 2 in, 2 out]
        n470 = property on="X mm/rev" class="DigNum (strict)"() -> ("Value"=w838:dbl)  [unwired: 2 in, 2 out]
        n471 = property on="Y mm/rev" class="DigNum (strict)"() -> ("Value"=w824:dbl)  [unwired: 2 in, 2 out]
        n472 = Multiply(x=w814, y=w811) -> (x*y=w806:dbl)
        n473 = Divide(x=w801, y=w800) -> (x/y=w799:dbl)
        n474 = Divide(x=w800, y=w809) -> (x/y=w807:dbl)
        n475 = Multiply(x=w838, y=w834) -> (x*y=w832:dbl)
        n476 = Divide(x=w793, y=w792) -> (x/y=w794:dbl)
        n477 = Divide(x=w792, y=w836) -> (x/y=w841:dbl)
        n478 = Multiply(x=w827, y=w824) -> (x*y=w820:dbl)
        n479 = Divide(x=w797, y=w796) -> (x/y=w795:dbl)
        n480 = Divide(x=w796, y=w798) -> (x/y=w821:dbl)
        n481 = Multiply(x=w811, y=w807) -> (x*y=w805:dbl)
        n482 = property on="X Scan length MV mm" class="DigNum (strict)"("Val(Sgnl)"=w832) -> ()  [unwired: 2 in, 2 out]
        n483 = Multiply(x=w841, y=w838) -> (x*y=w833:dbl)
        n484 = Multiply(x=w824, y=w821) -> (x*y=w819:dbl)
        n485 = property on="Z Scan length MV mm" class="DigNum (strict)"("Value"=w806) -> ()  [unwired: 2 in, 2 out]
        n486 = Absolute Value(x=w799) -> (abs(x)=→"Z Scan Duration":dbl)
        n487 = Absolute Value(x=w794) -> (abs(x)=→"X Scan Duration":dbl)
        n488 = property on="Y Scan length MV mm" class="DigNum (strict)"("Value"=w820) -> ()  [unwired: 2 in, 2 out]
        n489 = Absolute Value(x=w795) -> (abs(x)=→"Y Scan Duration":dbl)
        n490 = property on="Z Scan velocity MV mm/sec" class="DigNum (strict)"("Val(Sgnl)"=w805) -> ()  [unwired: 2 in, 2 out]
        n491 = property on="Y Scan velocity MV mm/sec" class="DigNum (strict)"("Val(Sgnl)"=w819) -> ()  [unwired: 2 in, 2 out]
        n492 = property on="X Scan velocity MV mm/sec" class="DigNum (strict)"("Value"=w833) -> ()  [unwired: 2 in, 2 out]
      }
      event "Y Move Set": Mouse Down {
        n493 = event-data() -> ()  [unwired: 1 in, 7 out]
        n494 = property on="Y steps/rev" class="DigNum (strict)"() -> ("Value"=w862:u32)  [unwired: 2 in, 2 out]
        n495 = property on="Y offset mm" class="DigNum (strict)"() -> ("Value"=w860:dbl)  [unwired: 2 in, 2 out]
        n496 = property on="Y Position SP mm" class="DigNum (strict)"() -> ("Value"=w859:dbl)  [unwired: 2 in, 2 out]
        n497 = property on="Y Velocity SP step/sec" class="DigNum (strict)"() -> ("Maximum"=w849:dbl)  [unwired: 2 in, 2 out]
        n498 = property on="Y Velocity SP step/sec" class="DigNum (strict)"() -> ("Minimum"=w848:dbl)  [unwired: 2 in, 2 out]
        n499 = Subtract(x=w859, y=w860) -> (x-y=w863:dbl)
        n500 = property on="Y Velocity SP mm/sec" class="DigNum (strict)"() -> ("Value"=w853:dbl)  [unwired: 2 in, 2 out]
        n501 = property on="Y mm/rev" class="DigNum (strict)"() -> ("Value"=w846:dbl)  [unwired: 2 in, 2 out]
        n502 = Divide(x=w863, y=w846) -> (x/y=w864:dbl)
        n503 = Divide(x=w853, y=w846) -> (x/y=w854:dbl)
        n504 = To Double Precision Float(number=w862) -> (double precision float=w847:dbl)
        n505 = Multiply(x=w864, y=w847) -> (x*y=w858:dbl)
        n506 = Multiply(x=w854, y=w847) -> (x*y=w851:dbl)
        n507 = property on="Y Step SP" class="DigNum (strict)"() -> ("Maximum"=w856:dbl)  [unwired: 2 in, 2 out]
        n508 = property on="Y Step SP" class="DigNum (strict)"() -> ("Minimum"=w855:dbl)  [unwired: 2 in, 2 out]
        n509 = In Range and Coerce(upper limit=w849, x=w851, lower limit=w848) -> (coerced(x)=w850:dbl)  [unwired: 1 out]
        n510 = To Long Integer(number=w850) -> (32bit integer=w852:i32)
        n511 = In Range and Coerce(upper limit=w856, x=w858, lower limit=w855) -> (coerced(x)=w857:dbl)  [unwired: 1 out]
        n512 = property on="Y Velocity SP step/sec" class="DigNum (strict)"("Val(Sgnl)"=w852) -> ()  [unwired: 2 in, 2 out]
        n513 = To Long Integer(number=w857) -> (32bit integer=w861:i32)
        n514 = property on="Y Step SP" class="DigNum (strict)"("Val(Sgnl)"=w861) -> ()  [unwired: 2 in, 2 out]
      }
      event "X Move Set": Mouse Down {
        n515 = event-data() -> ()  [unwired: 1 in, 7 out]
        n516 = property on="X steps/rev" class="DigNum (strict)"() -> ("Value"=w881:u32)  [unwired: 2 in, 2 out]
        n517 = property on="X offset mm" class="DigNum (strict)"() -> ("Value"=w879:dbl)  [unwired: 2 in, 2 out]
        n518 = property on="X Position SP mm" class="DigNum (strict)"() -> ("Value"=w878:dbl)  [unwired: 2 in, 2 out]
        n519 = property on="X Velocity SP step/sec" class="DigNum (strict)"() -> ("Maximum"=w868:dbl)  [unwired: 2 in, 2 out]
        n520 = property on="X Velocity SP step/sec" class="DigNum (strict)"() -> ("Minimum"=w867:dbl)  [unwired: 2 in, 2 out]
        n521 = Subtract(x=w878, y=w879) -> (x-y=w882:dbl)
        n522 = property on="X Velocity SP mm/sec" class="DigNum (strict)"() -> ("Value"=w872:dbl)  [unwired: 2 in, 2 out]
        n523 = property on="X mm/rev" class="DigNum (strict)"() -> ("Value"=w865:dbl)  [unwired: 2 in, 2 out]
        n524 = Divide(x=w882, y=w865) -> (x/y=w883:dbl)
        n525 = Divide(x=w872, y=w865) -> (x/y=w873:dbl)
        n526 = To Double Precision Float(number=w881) -> (double precision float=w866:dbl)
        n527 = Multiply(x=w883, y=w866) -> (x*y=w877:dbl)
        n528 = Multiply(x=w873, y=w866) -> (x*y=w870:dbl)
        n529 = property on="X Step SP" class="DigNum (strict)"() -> ("Maximum"=w875:dbl)  [unwired: 2 in, 2 out]
        n530 = property on="X Step SP" class="DigNum (strict)"() -> ("Minimum"=w874:dbl)  [unwired: 2 in, 2 out]
        n531 = In Range and Coerce(upper limit=w868, x=w870, lower limit=w867) -> (coerced(x)=w869:dbl)  [unwired: 1 out]
        n532 = To Long Integer(number=w869) -> (32bit integer=w871:i32)
        n533 = In Range and Coerce(upper limit=w875, x=w877, lower limit=w874) -> (coerced(x)=w876:dbl)  [unwired: 1 out]
        n534 = property on="X Velocity SP step/sec" class="DigNum (strict)"("Val(Sgnl)"=w871) -> ()  [unwired: 2 in, 2 out]
        n535 = To Long Integer(number=w876) -> (32bit integer=w880:i32)
        n536 = property on="X Step SP" class="DigNum (strict)"("Val(Sgnl)"=w880) -> ()  [unwired: 2 in, 2 out]
      }
      event "Z Move Set": Mouse Down {
        n537 = event-data() -> ()  [unwired: 1 in, 7 out]
        n538 = property on="Z steps/rev" class="DigNum (strict)"() -> ("Value"=w898:u32)  [unwired: 2 in, 2 out]
        n539 = property on="Z offset mm" class="DigNum (strict)"() -> ("Value"=w896:dbl)  [unwired: 2 in, 2 out]
        n540 = property on="Z Position SP mm" class="DigNum (strict)"() -> ("Value"=w895:dbl)  [unwired: 2 in, 2 out]
        n541 = property on="Z Velocity SP step/sec" class="DigNum (strict)"() -> ("Maximum"=w885:dbl)  [unwired: 2 in, 2 out]
        n542 = property on="Z Velocity SP step/sec" class="DigNum (strict)"() -> ("Minimum"=w884:dbl)  [unwired: 2 in, 2 out]
        n543 = Subtract(x=w895, y=w896) -> (x-y=w899:dbl)
        n544 = property on="Z Velocity SP mm/sec" class="DigNum (strict)"() -> ("Value"=w889:dbl)  [unwired: 2 in, 2 out]
        n545 = property on="Z mm/rev" class="DigNum (strict)"() -> ("Value"=w901:dbl)  [unwired: 2 in, 2 out]
        n546 = Divide(x=w899, y=w901) -> (x/y=w900:dbl)
        n547 = Divide(x=w889, y=w901) -> (x/y=w890:dbl)
        n548 = To Double Precision Float(number=w898) -> (double precision float=w902:dbl)
        n549 = Multiply(x=w900, y=w902) -> (x*y=w894:dbl)
        n550 = Multiply(x=w890, y=w902) -> (x*y=w887:dbl)
        n551 = property on="Z Step SP" class="DigNum (strict)"() -> ("Maximum"=w892:dbl)  [unwired: 2 in, 2 out]
        n552 = property on="Z Step SP" class="DigNum (strict)"() -> ("Minimum"=w891:dbl)  [unwired: 2 in, 2 out]
        n553 = In Range and Coerce(upper limit=w885, x=w887, lower limit=w884) -> (coerced(x)=w886:dbl)  [unwired: 1 out]
        n554 = To Long Integer(number=w886) -> (32bit integer=w888:i32)
        n555 = In Range and Coerce(upper limit=w892, x=w894, lower limit=w891) -> (coerced(x)=w893:dbl)  [unwired: 1 out]
        n556 = property on="Z Velocity SP step/sec" class="DigNum (strict)"("Val(Sgnl)"=w888) -> ()  [unwired: 2 in, 2 out]
        n557 = To Long Integer(number=w893) -> (32bit integer=w897:i32)
        n558 = property on="Z Step SP" class="DigNum (strict)"("Val(Sgnl)"=w897) -> ()  [unwired: 2 in, 2 out]
      }
      event "Y Scan set": Mouse Down {
        n559 = event-data() -> ()  [unwired: 1 in, 7 out]
        n560 = property on="Y steps/rev" class="DigNum (strict)"() -> ("Value"=w918:u32)  [unwired: 2 in, 2 out]
        n561 = To Double Precision Float(number=w918) -> (double precision float=w904:dbl)
        n562 = property on="Y mm/rev" class="DigNum (strict)"() -> ("Value"=w903:dbl)  [unwired: 2 in, 2 out]
        n563 = property on="Y Scan Length SP mm" class="DigNum (strict)"() -> ("Value"=w916:dbl)  [unwired: 2 in, 2 out]
        n564 = property on="Y Scan Velocity SP mm/sec" class="DigNum (strict)"() -> ("Value"=w910:dbl)  [unwired: 2 in, 2 out]
        n565 = property on="Y Scan Velocity SP steps/sec" class="DigNum (strict)"() -> ("Maximum"=w906:dbl)  [unwired: 2 in, 2 out]
        n566 = property on="Y Scan Velocity SP steps/sec" class="DigNum (strict)"() -> ("Minimum"=w905:dbl)  [unwired: 2 in, 2 out]
        n567 = Divide(x=w916, y=w903) -> (x/y=w919:dbl)
        n568 = Divide(x=w910, y=w903) -> (x/y=w911:dbl)
        n569 = Multiply(x=w919, y=w904) -> (x*y=w915:dbl)
        n570 = Multiply(x=w911, y=w904) -> (x*y=w908:dbl)
        n571 = property on="Y Step SP" class="DigNum (strict)"() -> ("Maximum"=w912:dbl)  [unwired: 2 in, 2 out]
        n572 = property on="Y Step SP" class="DigNum (strict)"() -> ("Minimum"=w913:dbl)  [unwired: 2 in, 2 out]
        n573 = In Range and Coerce(upper limit=w906, x=w908, lower limit=w905) -> (coerced(x)=w907:dbl)  [unwired: 1 out]
        n574 = To Long Integer(number=w907) -> (32bit integer=w909:i32)
        n575 = In Range and Coerce(upper limit=w912, x=w915, lower limit=w913) -> (coerced(x)=w914:dbl)  [unwired: 1 out]
        n576 = property on="Y Scan Velocity SP steps/sec" class="DigNum (strict)"("Val(Sgnl)"=w909) -> ()  [unwired: 2 in, 2 out]
        n577 = To Long Integer(number=w914) -> (32bit integer=w917:i32)
        n578 = property on="Y Scan Length SP steps" class="DigNum (strict)"("Val(Sgnl)"=w917) -> ()  [unwired: 2 in, 2 out]
      }
      event "X Scan set": Mouse Down {
        n579 = event-data() -> ()  [unwired: 1 in, 7 out]
        n580 = property on="X steps/rev" class="DigNum (strict)"() -> ("Value"=w935:u32)  [unwired: 2 in, 2 out]
        n581 = To Double Precision Float(number=w935) -> (double precision float=w921:dbl)
        n582 = property on="X mm/rev" class="DigNum (strict)"() -> ("Value"=w920:dbl)  [unwired: 2 in, 2 out]
        n583 = property on="X Scan Length SP mm" class="DigNum (strict)"() -> ("Value"=w933:dbl)  [unwired: 2 in, 2 out]
        n584 = property on="X Scan Velocity SP mm/sec" class="DigNum (strict)"() -> ("Value"=w927:dbl)  [unwired: 2 in, 2 out]
        n585 = property on="X Scan Velocity SP steps/sec" class="DigNum (strict)"() -> ("Maximum"=w923:dbl)  [unwired: 2 in, 2 out]
        n586 = property on="X Scan Velocity SP steps/sec" class="DigNum (strict)"() -> ("Minimum"=w922:dbl)  [unwired: 2 in, 2 out]
        n587 = Divide(x=w933, y=w920) -> (x/y=w936:dbl)
        n588 = Divide(x=w927, y=w920) -> (x/y=w928:dbl)
        n589 = Multiply(x=w936, y=w921) -> (x*y=w932:dbl)
        n590 = Multiply(x=w928, y=w921) -> (x*y=w925:dbl)
        n591 = property on="X Step SP" class="DigNum (strict)"() -> ("Maximum"=w929:dbl)  [unwired: 2 in, 2 out]
        n592 = property on="X Step SP" class="DigNum (strict)"() -> ("Minimum"=w930:dbl)  [unwired: 2 in, 2 out]
        n593 = In Range and Coerce(upper limit=w923, x=w925, lower limit=w922) -> (coerced(x)=w924:dbl)  [unwired: 1 out]
        n594 = To Long Integer(number=w924) -> (32bit integer=w926:i32)
        n595 = In Range and Coerce(upper limit=w929, x=w932, lower limit=w930) -> (coerced(x)=w931:dbl)  [unwired: 1 out]
        n596 = property on="X Scan Velocity SP steps/sec" class="DigNum (strict)"("Val(Sgnl)"=w926) -> ()  [unwired: 2 in, 2 out]
        n597 = To Long Integer(number=w931) -> (32bit integer=w934:i32)
        n598 = property on="X Scan Length SP steps" class="DigNum (strict)"("Val(Sgnl)"=w934) -> ()  [unwired: 2 in, 2 out]
      }
      event "Z Scan set": Mouse Down {
        n599 = event-data() -> ()  [unwired: 1 in, 7 out]
        n600 = property on="Z steps/rev" class="DigNum (strict)"() -> ("Value"=w952:u32)  [unwired: 2 in, 2 out]
        n601 = To Double Precision Float(number=w952) -> (double precision float=w938:dbl)
        n602 = property on="Z mm/rev" class="DigNum (strict)"() -> ("Value"=w937:dbl)  [unwired: 2 in, 2 out]
        n603 = property on="Z Scan Length SP mm" class="DigNum (strict)"() -> ("Value"=w950:dbl)  [unwired: 2 in, 2 out]
        n604 = property on="Z Scan Velocity SP mm/sec" class="DigNum (strict)"() -> ("Value"=w944:dbl)  [unwired: 2 in, 2 out]
        n605 = property on="Z Scan Velocity SP steps/sec" class="DigNum (strict)"() -> ("Maximum"=w940:dbl)  [unwired: 2 in, 2 out]
        n606 = property on="Z Scan Velocity SP steps/sec" class="DigNum (strict)"() -> ("Minimum"=w939:dbl)  [unwired: 2 in, 2 out]
        n607 = Divide(x=w950, y=w937) -> (x/y=w953:dbl)
        n608 = Divide(x=w944, y=w937) -> (x/y=w945:dbl)
        n609 = Multiply(x=w953, y=w938) -> (x*y=w949:dbl)
        n610 = Multiply(x=w945, y=w938) -> (x*y=w942:dbl)
        n611 = property on="Z Step SP" class="DigNum (strict)"() -> ("Maximum"=w946:dbl)  [unwired: 2 in, 2 out]
        n612 = property on="Z Step SP" class="DigNum (strict)"() -> ("Minimum"=w947:dbl)  [unwired: 2 in, 2 out]
        n613 = In Range and Coerce(upper limit=w940, x=w942, lower limit=w939) -> (coerced(x)=w941:dbl)  [unwired: 1 out]
        n614 = To Long Integer(number=w941) -> (32bit integer=w943:i32)
        n615 = In Range and Coerce(upper limit=w946, x=w949, lower limit=w947) -> (coerced(x)=w948:dbl)  [unwired: 1 out]
        n616 = property on="Z Scan Velocity SP steps/sec" class="DigNum (strict)"("Val(Sgnl)"=w943) -> ()  [unwired: 2 in, 2 out]
        n617 = To Long Integer(number=w948) -> (32bit integer=w951:i32)
        n618 = property on="Z Scan Length SP steps" class="DigNum (strict)"("Val(Sgnl)"=w951) -> ()  [unwired: 2 in, 2 out]
      }
      event "Y Go": Mouse Up {
        n619 = event-data() -> ()  [unwired: 1 in, 7 out]
        n620 = flat-sequence {
          tunnel: w960 -> [w970]
          tunnel: w961 -> [w971]
          tunnel: [w971] -> w957
          tunnel: [w970] -> w956
          tunnel: [w974] -> w959
          tunnel: [w973] -> w958
          tunnel: w957 -> [w976]
          tunnel: w956 -> [w975]
          tunnel: [w997] -> w963
          tunnel: [w992] -> w962
          tunnel: w959 -> [w996]
          tunnel: w958 -> [w995]
          tunnel: [w991] -> w955
          tunnel: [w1008] -> w965
          tunnel: [w1003] -> w964
          tunnel: w963 -> [w1006]
          tunnel: w962 -> [w1007]
          tunnel: w955 -> [w1004]
          tunnel: [w1004] -> w954
          tunnel: [w1011] -> w966
          tunnel: [w1014] -> w967
          tunnel: w965 -> [w1013]
          tunnel: w964 -> [w1012]
          tunnel: w954 -> [w1015]
          frame #0 {
            n621 = property on="Scan Go" class="Bool"("DisabledEnum"=T2."Disabled and Grayed Out" ("Disabled")) -> ()  [unwired: 2 in, 2 out]
            n622 = property on="Y Go" class="Bool"("DisabledEnum"=T2."Disabled and Grayed Out" ("Disabled")) -> ()  [unwired: 2 in, 2 out]
          }
          frame #1 {
            n623 = property on="Y Step SP" class="DigNum (strict)"() -> ("Value"=w984:i32)  [unwired: 2 in, 2 out]
            n624 = property on="Y Step PV" class="DigNum (strict)"() -> ("Value"=w983:i32)  [unwired: 2 in, 2 out]
            n625 = property on="Y Backlash" class="DigNum (strict)"() -> ("Value"=w972:i32)  [unwired: 2 in, 2 out]
            n626 = Subtract(x=w984, y=w983) -> (x-y=w982:i32)
            n627 = Sign(1:w972) -> (0:w980:i32)
            n628 = Sign(1:w982) -> (0:w981:i32)
            n629 = Multiply(x=w981, y=w980) -> (x*y=w979:i32)
            n630 = Equal?(x=w979, y=1) -> (x = y?=w977:bool)
            n631 = case shown="False" w977 {
              tunnel: w976 -> [w987 w989]
              tunnel: w975 -> [w986 w988]
              tunnel: [w986 w988] -> w974
              tunnel: [w987 w989] -> w973
              frame False {
                n632 = property on="Y Backlash corr" class="Bool (strict)"("Val(Sgnl)"=FALSE ("Value (Signaling)")) -> ()  [unwired: 2 in, 2 out]
              }
              frame True {
                n633 = property on="Y Backlash corr" class="Bool (strict)"("Val(Sgnl)"=TRUE ("Value (Signaling)")) -> ()  [unwired: 2 in, 2 out]
              }
            }
          }
          frame #2 {
            w991 = 0.1 ("Delay Time (s)")
            # "Velocity Setting"
            n634 = property on="Y Velocity SP step/sec" class="DigNum (strict)"() -> ("Value"=w1000:i32)  [unwired: 2 in, 2 out]
            n635 = Number To Decimal String(number=w1000) -> ()  [unwired: 1 in, 1 out]
            n636 = property on="Y steps/rev" class="DigNum (strict)"() -> ("Value"=w999:u32)  [unwired: 2 in, 2 out]
            n637 = Divide(x=w1000, y=w999) -> (x/y=w1001:dbl)
            n638 = Number To Fractional String(number=w1001) -> (F-format string=w994:string)  [unwired: 3 in]
            n639 = call "Applied Send Command.vi"("error in (no error)"=w996, "Extra"=w994, "Command"=T1."Velocity Setting", "VISA resource name"=w995) -> ("error out"=w993:errorcluster, "VISA resource name out"=w997:refnum<visa-resource-name>)  [unwired: 3 in, 1 out]
            n640 = call "Time Delay22"("error in (no error)"=w993, "Delay Time (s)"=w991) -> ("error out"=w992:errorcluster)  [unwired: 9 in]
          }
          frame #3 {
            # "Move to Abs Position"
            n641 = property on="Y Step SP" class="DigNum (strict)"() -> ("Value"=w1010:i32)  [unwired: 2 in, 2 out]
            n642 = Number To Decimal String(number=w1010) -> (decimal integer string=w1005:string)  [unwired: 1 in]
            n643 = call "Applied Send Command.vi"("error in (no error)"=w1007, "Extra"=w1005, "Command"=T1."Distance or Position", "VISA resource name"=w1006) -> ("error out"=w1002:errorcluster, "VISA resource name out"=w1008:refnum<visa-resource-name>)  [unwired: 3 in, 1 out]
            n644 = call "Time Delay"("error in (no error)"=w1002, "Delay Time (s)"=w1004) -> ("error out"=w1003:errorcluster)  [unwired: 9 in]
          }
          frame #4 {
            n645 = call "Applied Send Command.vi"("error in (no error)"=w1012, "Command"=T1."Feed to Position", "VISA resource name"=w1013) -> ("error out"=w1016:errorcluster, "VISA resource name out"=w1014:refnum<visa-resource-name>)  [unwired: 4 in, 1 out]
            n646 = call "Time Delay23"("error in (no error)"=w1016, "Delay Time (s)"=w1015) -> ("error out"=w1011:errorcluster)  [unwired: 9 in]
          }
        }
      }
      event "Z Go": Mouse Up {
        n647 = event-data() -> ()  [unwired: 1 in, 7 out]
        n648 = flat-sequence {
          tunnel: w1022 -> [w1034]
          tunnel: w1023 -> [w1035]
          tunnel: [w1035] -> w1025
          tunnel: [w1034] -> w1024
          tunnel: [w1038] -> w1027
          tunnel: [w1037] -> w1026
          tunnel: w1025 -> [w1040]
          tunnel: w1024 -> [w1039]
          tunnel: [w1058] -> w1029
          tunnel: [w1056] -> w1028
          tunnel: w1027 -> [w1059]
          tunnel: w1026 -> [w1060]
          tunnel: [w1055] -> w1019
          tunnel: [w1069] -> w1031
          tunnel: [w1068] -> w1030
          tunnel: w1029 -> [w1070]
          tunnel: w1028 -> [w1072]
          tunnel: w1019 -> [w1066]
          tunnel: [w1066] -> w1018
          tunnel: [w1081] -> w1021
          tunnel: [w1077] -> w1020
          tunnel: w1031 -> [w1078]
          tunnel: w1030 -> [w1075]
          tunnel: w1018 -> [w1080]
          frame #0 {
            n649 = property on="Scan Go" class="Bool"("DisabledEnum"=T2."Disabled and Grayed Out" ("Disabled")) -> ()  [unwired: 2 in, 2 out]
            n650 = property on="Z Go" class="Bool"("DisabledEnum"=T2."Disabled and Grayed Out" ("Disabled")) -> ()  [unwired: 2 in, 2 out]
          }
          frame #1 {
            n651 = property on="Z Step SP" class="DigNum (strict)"() -> ("Value"=w1048:i32)  [unwired: 2 in, 2 out]
            n652 = property on="Z Step PV" class="DigNum (strict)"() -> ("Value"=w1047:i32)  [unwired: 2 in, 2 out]
            n653 = property on="Z Backlash" class="DigNum (strict)"() -> ("Value"=w1036:i32)  [unwired: 2 in, 2 out]
            n654 = Subtract(x=w1048, y=w1047) -> (x-y=w1046:i32)
            n655 = Sign(1:w1036) -> (0:w1044:i32)
            n656 = Sign(1:w1046) -> (0:w1045:i32)
            n657 = Multiply(x=w1045, y=w1044) -> (x*y=w1043:i32)
            n658 = Equal?(x=w1043, y=1) -> (x = y?=w1041:bool)
            n659 = case shown="True" w1041 {
              tunnel: w1040 -> [w1051 w1053]
              tunnel: w1039 -> [w1050 w1052]
              tunnel: [w1050 w1052] -> w1038
              tunnel: [w1051 w1053] -> w1037
              frame False {
                n660 = property on="Z Backlash corr" class="Bool (strict)"("Val(Sgnl)"=FALSE ("Value (Signaling)")) -> ()  [unwired: 2 in, 2 out]
              }
              frame True {
                n661 = property on="Z Backlash corr" class="Bool (strict)"("Val(Sgnl)"=TRUE ("Value (Signaling)")) -> ()  [unwired: 2 in, 2 out]
              }
            }
          }
          frame #2 {
            w1055 = 0.1 ("Delay Time (s)")
            n662 = property on="Z Velocity SP step/sec" class="DigNum (strict)"() -> ("Value"=w1062:i32)  [unwired: 2 in, 2 out]
            n663 = property on="Z steps/rev" class="DigNum (strict)"() -> ("Value"=w1061:u32)  [unwired: 2 in, 2 out]
            n664 = Divide(x=w1062, y=w1061) -> (x/y=w1063:dbl)
            n665 = Number To Fractional String(number=w1063) -> (F-format string=w1064:string)  [unwired: 3 in]
            n666 = call "Applied Send Command.vi"("error in (no error)"=w1059, "Extra"=w1064, "Command"=T1."Velocity Setting", "VISA resource name"=w1060) -> ("error out"=w1057:errorcluster, "VISA resource name out"=w1058:refnum<visa-resource-name>)  [unwired: 3 in, 1 out]
            n667 = call "Time Delay52"("error in (no error)"=w1057, "Delay Time (s)"=w1055) -> ("error out"=w1056:errorcluster)  [unwired: 9 in]
          }
          frame #3 {
            # "Move to Abs Position"
            n668 = property on="Z Step SP" class="DigNum (strict)"() -> ("Value"=w1074:i32)  [unwired: 2 in, 2 out]
            n669 = Number To Decimal String(number=w1074) -> (decimal integer string=w1071:string)  [unwired: 1 in]
            n670 = call "Applied Send Command.vi"("error in (no error)"=w1072, "Extra"=w1071, "Command"=T1."Distance or Position", "VISA resource name"=w1070) -> ("error out"=w1067:errorcluster, "VISA resource name out"=w1069:refnum<visa-resource-name>)  [unwired: 3 in, 1 out]
            n671 = call "Time Delay51"("error in (no error)"=w1067, "Delay Time (s)"=w1066) -> ("error out"=w1068:errorcluster)  [unwired: 9 in]
          }
          frame #4 {
            n672 = call "Applied Send Command.vi"("error in (no error)"=w1075, "Command"=T1."Feed to Position", "VISA resource name"=w1078) -> ("error out"=w1076:errorcluster, "VISA resource name out"=w1077:refnum<visa-resource-name>)  [unwired: 4 in, 1 out]
            n673 = call "Time Delay28"("error in (no error)"=w1076, "Delay Time (s)"=w1080) -> ("error out"=w1081:errorcluster)  [unwired: 9 in]
          }
        }
      }
      event "X Go": Mouse Up {
        n674 = event-data() -> ()  [unwired: 1 in, 7 out]
        n675 = flat-sequence {
          tunnel: [w1097] -> w1093
          tunnel: [w1096] -> w1092
          tunnel: w1091 -> [w1097]
          tunnel: w1090 -> [w1096]
          tunnel: [w1102] -> w1095
          tunnel: [w1101] -> w1094
          tunnel: w1093 -> [w1104]
          tunnel: w1092 -> [w1103]
          tunnel: [w1123] -> w1087
          tunnel: [w1120] -> w1085
          tunnel: w1095 -> [w1124]
          tunnel: w1094 -> [w1125]
          tunnel: [w1119] -> w1083
          tunnel: w1087 -> [w1132]
          tunnel: [w1131] -> w1086
          tunnel: w1085 -> [w1133]
          tunnel: [w1134] -> w1084
          tunnel: w1083 -> [w1130]
          tunnel: [w1130] -> w1082
          tunnel: w1086 -> [w1144]
          tunnel: w1084 -> [w1143]
          tunnel: [w1142] -> w1089
          tunnel: [w1141] -> w1088
          tunnel: w1082 -> [w1139]
          frame #0 {
            n676 = property on="Scan Go" class="Bool"("DisabledEnum"=T2."Disabled and Grayed Out" ("Disabled")) -> ()  [unwired: 2 in, 2 out]
            n677 = property on="X Go" class="Bool"("DisabledEnum"=T2."Disabled and Grayed Out" ("Disabled")) -> ()  [unwired: 2 in, 2 out]
          }
          frame #1 {
            n678 = property on="X Step SP" class="DigNum (strict)"() -> ("Value"=w1112:i32)  [unwired: 2 in, 2 out]
            n679 = property on="X Step PV" class="DigNum (strict)"() -> ("Value"=w1111:i32)  [unwired: 2 in, 2 out]
            n680 = property on="X Backlash" class="DigNum (strict)"() -> ("Value"=w1100:i32)  [unwired: 2 in, 2 out]
            n681 = Subtract(x=w1112, y=w1111) -> (x-y=w1110:i32)
            n682 = Sign(1:w1100) -> (0:w1108:i32)
            n683 = Sign(1:w1110) -> (0:w1109:i32)
            n684 = Multiply(x=w1109, y=w1108) -> (x*y=w1107:i32)
            n685 = Equal?(x=w1107, y=1) -> (x = y?=w1105:bool)
            n686 = case shown="True" w1105 {
              tunnel: w1104 -> [w1115 w1117]
              tunnel: w1103 -> [w1114 w1116]
              tunnel: [w1114 w1116] -> w1102
              tunnel: [w1115 w1117] -> w1101
              frame False {
                n687 = property on="X Backlash corr" class="Bool (strict)"("Val(Sgnl)"=FALSE ("Value (Signaling)")) -> ()  [unwired: 2 in, 2 out]
              }
              frame True {
                n688 = property on="X Backlash corr" class="Bool (strict)"("Val(Sgnl)"=TRUE ("Value (Signaling)")) -> ()  [unwired: 2 in, 2 out]
              }
            }
          }
          frame #2 {
            w1119 = 0.1 ("Delay Time (s)")
            n689 = property on="X Velocity SP step/sec" class="DigNum (strict)"() -> ("Value"=w1122:i32)  [unwired: 2 in, 2 out]
            n690 = property on="X steps/rev" class="DigNum (strict)"() -> ("Value"=w1126:u32)  [unwired: 2 in, 2 out]
            n691 = Divide(x=w1122, y=w1126) -> (x/y=w1127:dbl)
            n692 = Number To Fractional String(number=w1127) -> (F-format string=w1128:string)  [unwired: 3 in]
            n693 = call "Applied Send Command.vi"("error in (no error)"=w1124, "Extra"=w1128, "Command"=T1."Velocity Setting", "VISA resource name"=w1125) -> ("error out"=w1121:errorcluster, "VISA resource name out"=w1123:refnum<visa-resource-name>)  [unwired: 3 in, 1 out]
            n694 = call "Time Delay14"("error in (no error)"=w1121, "Delay Time (s)"=w1119) -> ("error out"=w1120:errorcluster)  [unwired: 9 in]
          }
          frame #3 {
            # "Distance/Position"
            n695 = property on="X Step SP" class="DigNum (strict)"() -> ("Value"=w1135:i32)  [unwired: 2 in, 2 out]
            n696 = Number To Decimal String(number=w1135) -> (decimal integer string=w1137:string)  [unwired: 1 in]
            n697 = call "Applied Send Command.vi"("error in (no error)"=w1133, "Extra"=w1137, "Command"=T1."Distance or Position", "VISA resource name"=w1132) -> ("error out"=w1136:errorcluster, "VISA resource name out"=w1131:refnum<visa-resource-name>)  [unwired: 3 in, 1 out]
            n698 = call "Time Delay31"("error in (no error)"=w1136, "Delay Time (s)"=w1130) -> ("error out"=w1134:errorcluster)  [unwired: 9 in]
          }
          frame #4 {
            # "Feed to Position"
            n699 = call "Applied Send Command.vi"("error in (no error)"=w1143, "Command"=T1."Feed to Position", "VISA resource name"=w1144) -> ("error out"=w1140:errorcluster, "VISA resource name out"=w1142:refnum<visa-resource-name>)  [unwired: 4 in, 1 out]
            n700 = call "Time Delay15"("error in (no error)"=w1140, "Delay Time (s)"=w1139) -> ("error out"=w1141:errorcluster)  [unwired: 9 in]
          }
        }
      }
      event "X Scan OK": Mouse Up {
        n701 = event-data() -> ()  [unwired: 1 in, 7 out]
        n702 = flat-sequence {
          tunnel: [w1161] -> w1153
          tunnel: [w1172] -> w1152
          tunnel: w1151 -> [w1169]
          tunnel: w1150 -> [w1168]
          tunnel: w1153 -> [w1179]
          tunnel: w1152 -> [w1178]
          tunnel: [w1179] -> w1147
          tunnel: [w1178] -> w1146
          tunnel: [w1181] -> w1148
          tunnel: [w1182] -> w1149
          tunnel: w1147 -> [w1182]
          tunnel: w1146 -> [w1181]
          frame #0 {
            # "VELOCITY"
            n703 = property on="X steps/rev" class="DigNum (strict)"() -> ("Value"=w1154:u32)  [unwired: 2 in, 2 out]
            n704 = property on="X Scan Velocity SP steps/sec" class="DigNum (strict)"() -> ("Value"=w1155:i32)  [unwired: 2 in, 2 out]
            n705 = Divide(x=w1155, y=w1154) -> (x/y=w1156:dbl)
            n706 = Number To Fractional String(number=w1156) -> (F-format string=w1170:string)  [unwired: 3 in]
            n707 = call "Applied Send Command.vi"("error in (no error)"=w1168, "Extra"=w1170, "Command"=T1."Velocity Setting", "VISA resource name"=w1169) -> ("error out"=w1157:errorcluster, "VISA resource name out"=w1158:refnum<visa-resource-name>)  [unwired: 3 in, 1 out]
            n708 = call "Time Delay9"("error in (no error)"=w1157) -> ("error out"=w1159:errorcluster)  [unwired: 10 in]
            n709 = call "Applied Send Command.vi"("error in (no error)"=w1159, "Extra"="", "Command"=T1."Velocity Setting", "VISA resource name"=w1158) -> ("error out"=w1160:errorcluster, "read buffer"=w1165:string, "VISA resource name out"=w1161:refnum<visa-resource-name>)  [unwired: 3 in]
            n710 = call "Time Delay10"("error in (no error)"=w1160) -> ("error out"=w1172:errorcluster)  [unwired: 10 in]
            n711 = Fract/Exp String To Number(string=w1165, offset=3) -> (number=w1163:dbl)  [unwired: 2 in, 1 out]
            n712 = Multiply(x=w1163, y=w1154) -> (x*y=w1162:dbl)
            n713 = property on="X velocity PV step/sec" class="DigNum (strict)"("Val(Sgnl)"=w1162) -> ()  [unwired: 2 in, 2 out]
          }
          frame #1 {
            n714 = property on="X Scan" class="Bool (strict)"("Val(Sgnl)"=TRUE ("Slew Ready 2")) -> ()  [unwired: 2 in, 2 out]
            n715 = property on="Scan Cancel" class="Bool"("DisabledEnum"=T2."Enabled" ("Disabled")) -> ()  [unwired: 2 in, 2 out]
            n716 = property on="Scan Go" class="Bool"("DisabledEnum"=T2."Enabled" ("Disabled")) -> ()  [unwired: 2 in, 2 out]
            n717 = property on="X Scan Length SP steps" class="DigNum (strict)"("DisabledEnum"=T2."Disabled and Grayed Out" ("Disabled")) -> ()  [unwired: 2 in, 2 out]
            n718 = property on="X Scan Velocity SP steps/sec" class="DigNum (strict)"("DisabledEnum"=T2."Disabled and Grayed Out" ("Disabled")) -> ()  [unwired: 2 in, 2 out]
          }
          frame #2 {
            n719 = property on="X Go" class="Bool"("DisabledEnum"=T2."Disabled and Grayed Out" ("Disabled")) -> ()  [unwired: 2 in, 2 out]
          }
        }
      }
      event "Y Scan OK": Mouse Up {
        n720 = event-data() -> ()  [unwired: 1 in, 7 out]
        n721 = flat-sequence {
          tunnel: w1190 -> [w1202]
          tunnel: w1189 -> [w1203]
          tunnel: [w1193] -> w1187
          tunnel: [w1209] -> w1186
          tunnel: w1187 -> [w1216]
          tunnel: w1186 -> [w1215]
          tunnel: [w1216] -> w1184
          tunnel: [w1215] -> w1183
          tunnel: [w1218] -> w1188
          tunnel: [w1219] -> w1185
          tunnel: w1184 -> [w1219]
          tunnel: w1183 -> [w1218]
          frame #0 {
            # "VELOCITY"
            n722 = property on="Y Scan Velocity SP steps/sec" class="DigNum (strict)"() -> ("Value"=w1205:i32)  [unwired: 2 in, 2 out]
            n723 = property on="Y steps/rev" class="DigNum (strict)"() -> ("Value"=w1196:u32)  [unwired: 2 in, 2 out]
            n724 = Divide(x=w1205, y=w1196) -> (x/y=w1206:dbl)
            n725 = Number To Fractional String(number=w1206) -> (F-format string=w1207:string)  [unwired: 3 in]
            n726 = call "Applied Send Command.vi"("error in (no error)"=w1202, "Extra"=w1207, "Command"=T1."Velocity Setting", "VISA resource name"=w1203) -> ("error out"=w1204:errorcluster, "VISA resource name out"=w1194:refnum<visa-resource-name>)  [unwired: 3 in, 1 out]
            n727 = call "Time Delay5"("error in (no error)"=w1204) -> ("error out"=w1195:errorcluster)  [unwired: 10 in]
            n728 = call "Applied Send Command.vi"("error in (no error)"=w1195, "Extra"="", "Command"=T1."Velocity Setting", "VISA resource name"=w1194) -> ("error out"=w1192:errorcluster, "read buffer"=w1199:string, "VISA resource name out"=w1193:refnum<visa-resource-name>)  [unwired: 3 in]
            n729 = Fract/Exp String To Number(string=w1199, offset=3) -> (number=w1198:dbl)  [unwired: 2 in, 1 out]
            n730 = call "Time Delay6"("error in (no error)"=w1192) -> ("error out"=w1209:errorcluster)  [unwired: 10 in]
            n731 = Multiply(x=w1198, y=w1196) -> (x*y=w1197:dbl)
            n732 = property on="Y velocity PV step/sec" class="DigNum (strict)"("Val(Sgnl)"=w1197) -> ()  [unwired: 2 in, 2 out]
          }
          frame #1 {
            n733 = property on="Y Scan" class="Bool (strict)"("Val(Sgnl)"=TRUE ("Slew Ready 2")) -> ()  [unwired: 2 in, 2 out]
            n734 = property on="Scan Cancel" class="Bool"("DisabledEnum"=T2."Enabled" ("Disabled")) -> ()  [unwired: 2 in, 2 out]
            n735 = property on="Scan Go" class="Bool"("DisabledEnum"=T2."Enabled" ("Disabled")) -> ()  [unwired: 2 in, 2 out]
            n736 = property on="Y Scan Length SP steps" class="DigNum (strict)"("DisabledEnum"=T2."Disabled and Grayed Out" ("Disabled")) -> ()  [unwired: 2 in, 2 out]
            n737 = property on="Y Scan Velocity SP steps/sec" class="DigNum (strict)"("DisabledEnum"=T2."Disabled and Grayed Out" ("Disabled")) -> ()  [unwired: 2 in, 2 out]
          }
          frame #2 {
            n738 = property on="Y Go" class="Bool"("DisabledEnum"=T2."Disabled and Grayed Out" ("Disabled")) -> ()  [unwired: 2 in, 2 out]
          }
        }
      }
      event "Z Scan OK": Mouse Up {
        n739 = event-data() -> ()  [unwired: 1 in, 7 out]
        n740 = flat-sequence {
          tunnel: [w1232] -> w1227
          tunnel: [w1246] -> w1226
          tunnel: w1223 -> [w1228]
          tunnel: w1222 -> [w1229]
          tunnel: w1227 -> [w1253]
          tunnel: w1226 -> [w1252]
          tunnel: [w1253] -> w1225
          tunnel: [w1252] -> w1224
          tunnel: [w1255] -> w1221
          tunnel: [w1256] -> w1220
          tunnel: w1225 -> [w1256]
          tunnel: w1224 -> [w1255]
          frame #0 {
            # "VELOCITY"
            n741 = property on="Z Scan Velocity SP steps/sec" class="DigNum (strict)"() -> ("Value"=w1242:i32)  [unwired: 2 in, 2 out]
            n742 = property on="Z steps/rev" class="DigNum (strict)"() -> ("Value"=w1235:u32)  [unwired: 2 in, 2 out]
            n743 = Divide(x=w1242, y=w1235) -> (x/y=w1243:dbl)
            n744 = Number To Fractional String(number=w1243) -> (F-format string=w1244:string)  [unwired: 3 in]
            n745 = call "Applied Send Command.vi"("error in (no error)"=w1229, "Extra"=w1244, "Command"=T1."Velocity Setting", "VISA resource name"=w1228) -> ("error out"=w1241:errorcluster, "VISA resource name out"=w1231:refnum<visa-resource-name>)  [unwired: 3 in, 1 out]
            n746 = call "Time Delay24"("error in (no error)"=w1241) -> ("error out"=w1230:errorcluster)  [unwired: 10 in]
            n747 = call "Applied Send Command.vi"("error in (no error)"=w1230, "Extra"="", "Command"=T1."Velocity Setting", "VISA resource name"=w1231) -> ("error out"=w1233:errorcluster, "read buffer"=w1238:string, "VISA resource name out"=w1232:refnum<visa-resource-name>)  [unwired: 3 in]
            n748 = call "Time Delay25"("error in (no error)"=w1233) -> ("error out"=w1246:errorcluster)  [unwired: 10 in]
            n749 = Fract/Exp String To Number(string=w1238, offset=3) -> (number=w1237:dbl)  [unwired: 2 in, 1 out]
            n750 = Multiply(x=w1237, y=w1235) -> (x*y=w1234:dbl)
            n751 = property on="Z  velocity PV step/sec" class="DigNum (strict)"("Val(Sgnl)"=w1234) -> ()  [unwired: 2 in, 2 out]
          }
          frame #1 {
            n752 = property on="Z Scan" class="Bool (strict)"("Val(Sgnl)"=TRUE ("Slew Ready 2")) -> ()  [unwired: 2 in, 2 out]
            n753 = property on="Scan Cancel" class="Bool"("DisabledEnum"=T2."Enabled" ("Disabled")) -> ()  [unwired: 2 in, 2 out]
            n754 = property on="Scan Go" class="Bool"("DisabledEnum"=T2."Enabled" ("Disabled")) -> ()  [unwired: 2 in, 2 out]
            n755 = property on="Z Scan Length SP steps" class="DigNum (strict)"("DisabledEnum"=T2."Disabled and Grayed Out" ("Disabled")) -> ()  [unwired: 2 in, 2 out]
            n756 = property on="Z Scan Velocity SP steps/sec" class="DigNum (strict)"("DisabledEnum"=T2."Disabled and Grayed Out" ("Disabled")) -> ()  [unwired: 2 in, 2 out]
          }
          frame #2 {
            n757 = property on="Z Go" class="Bool"("DisabledEnum"=T2."Disabled and Grayed Out" ("Disabled")) -> ()  [unwired: 2 in, 2 out]
          }
        }
      }
      event Application Instance Close? {
        n758 = event-data() -> ()  [unwired: 1 in, 4 out]
        n759 = event-data() -> ()  [unwired: 3 in, 1 out]
      }
      event "Stop": Mouse Down {
        n760 = event-data() -> ()  [unwired: 1 in, 7 out]
        n761 = flat-sequence {
          tunnel: [w1278] -> w1266
          tunnel: [w1277] -> w1265
          tunnel: w1264 -> [w1279]
          tunnel: w1263 -> [w1276]
          frame #0 {
            n762 = call "Applied Send Command.vi"("error in (no error)"=w1276, "Command"=T1."Stop", "VISA resource name"=w1279) -> ("error out"=w1277:errorcluster, "VISA resource name out"=w1278:refnum<visa-resource-name>)  [unwired: 4 in, 1 out]
          }
        }
        n763 = flat-sequence {
          tunnel: w1270 -> [w1282]
          tunnel: w1269 -> [w1281]
          tunnel: [w1283] -> w1268
          tunnel: [w1284] -> w1267
          frame #0 {
            n764 = call "Applied Send Command.vi"("error in (no error)"=w1281, "Command"=T1."Stop", "VISA resource name"=w1282) -> ("error out"=w1284:errorcluster, "VISA resource name out"=w1283:refnum<visa-resource-name>)  [unwired: 4 in, 1 out]
          }
        }
        n765 = flat-sequence {
          tunnel: [w1273] -> w1260
          tunnel: [w1274] -> w1259
          tunnel: w1262 -> [w1271]
          tunnel: w1261 -> [w1272]
          frame #0 {
            n766 = call "Applied Send Command.vi"("error in (no error)"=w1272, "Command"=T1."Stop", "VISA resource name"=w1271) -> ("error out"=w1274:errorcluster, "VISA resource name out"=w1273:refnum<visa-resource-name>)  [unwired: 4 in, 1 out]
          }
        }
      }
      event "Scan Cancel": Mouse Down {
        n767 = event-data() -> ()  [unwired: 1 in, 7 out]
        n768 = flat-sequence {
          tunnel: w1295 -> [w1320]
          tunnel: w1294 -> [w1319]
          tunnel: [w1322] -> w1297
          tunnel: [w1321] -> w1296
          tunnel: [w1330] -> w1292
          tunnel: [w1331] -> w1293
          tunnel: w1297 -> [w1331]
          tunnel: w1296 -> [w1330]
          frame #0 {
            n769 = call "Applied Send Command.vi"("error in (no error)"=w1319, "Command"=T1."Stop", "VISA resource name"=w1320) -> ("error out"=w1321:errorcluster, "VISA resource name out"=w1322:refnum<visa-resource-name>)  [unwired: 4 in, 1 out]
          }
          frame #1 {
            n770 = property on="X Scan" class="Bool (strict)"("Value"=FALSE ("Slew Ready")) -> ()  [unwired: 2 in, 2 out]
            n771 = property on="X Scan set" class="Bool"("DisabledEnum"=T2."Enabled" ("Disabled")) -> ()  [unwired: 2 in, 2 out]
            n772 = property on="X Scan Velocity SP steps/sec" class="DigNum (strict)"("DisabledEnum"=T2."Enabled" ("Disabled")) -> ()  [unwired: 2 in, 2 out]
            n773 = property on="X Scan Length SP steps" class="DigNum (strict)"("DisabledEnum"=T2."Enabled" ("Disabled")) -> ()  [unwired: 2 in, 2 out]
            n774 = property on="X Go" class="Bool"("DisabledEnum"=T2."Enabled" ("Disabled")) -> ()  [unwired: 2 in, 2 out]
            n775 = property on="X Scan OK" class="Bool"("DisabledEnum"=T2."Enabled" ("Disabled")) -> ()  [unwired: 2 in, 2 out]
          }
        }
        n776 = flat-sequence {
          tunnel: w1303 -> [w1333]
          tunnel: w1302 -> [w1332]
          tunnel: [w1335] -> w1299
          tunnel: [w1334] -> w1298
          tunnel: [w1343] -> w1304
          tunnel: [w1344] -> w1305
          tunnel: w1299 -> [w1344]
          tunnel: w1298 -> [w1343]
          frame #0 {
            n777 = call "Applied Send Command.vi"("error in (no error)"=w1332, "Command"=T1."Stop", "VISA resource name"=w1333) -> ("error out"=w1334:errorcluster, "VISA resource name out"=w1335:refnum<visa-resource-name>)  [unwired: 4 in, 1 out]
          }
          frame #1 {
            n778 = property on="Y Scan" class="Bool (strict)"("Value"=FALSE ("Slew Ready")) -> ()  [unwired: 2 in, 2 out]
            n779 = property on="Y Go" class="Bool"("DisabledEnum"=T2."Enabled" ("Disabled")) -> ()  [unwired: 2 in, 2 out]
            n780 = property on="Y Scan Velocity SP steps/sec" class="DigNum (strict)"("DisabledEnum"=T2."Enabled" ("Disabled")) -> ()  [unwired: 2 in, 2 out]
            n781 = property on="Y Scan set" class="Bool"("DisabledEnum"=T2."Enabled" ("Disabled")) -> ()  [unwired: 2 in, 2 out]
            n782 = property on="Y Scan OK" class="Bool"("DisabledEnum"=T2."Enabled" ("Disabled")) -> ()  [unwired: 2 in, 2 out]
            n783 = property on="Y Scan Length SP steps" class="DigNum (strict)"("DisabledEnum"=T2."Enabled" ("Disabled")) -> ()  [unwired: 2 in, 2 out]
          }
        }
        n784 = flat-sequence {
          tunnel: [w1309] -> w1291
          tunnel: [w1308] -> w1290
          tunnel: w1289 -> [w1307]
          tunnel: w1288 -> [w1306]
          tunnel: [w1317] -> w1286
          tunnel: [w1318] -> w1287
          tunnel: w1291 -> [w1318]
          tunnel: w1290 -> [w1317]
          frame #0 {
            n785 = call "Applied Send Command.vi"("error in (no error)"=w1306, "Command"=T1."Stop", "VISA resource name"=w1307) -> ("error out"=w1308:errorcluster, "VISA resource name out"=w1309:refnum<visa-resource-name>)  [unwired: 4 in, 1 out]
          }
          frame #1 {
            n786 = property on="Z Scan" class="Bool (strict)"("Value"=FALSE ("Slew Ready")) -> ()  [unwired: 2 in, 2 out]
            n787 = property on="Z Scan set" class="Bool"("DisabledEnum"=T2."Enabled" ("Disabled")) -> ()  [unwired: 2 in, 2 out]
            n788 = property on="Z Scan Velocity SP steps/sec" class="DigNum (strict)"("DisabledEnum"=T2."Enabled" ("Disabled")) -> ()  [unwired: 2 in, 2 out]
            n789 = property on="Z Scan Length SP steps" class="DigNum (strict)"("DisabledEnum"=T2."Enabled" ("Disabled")) -> ()  [unwired: 2 in, 2 out]
            n790 = property on="Z Go" class="Bool"("DisabledEnum"=T2."Enabled" ("Disabled")) -> ()  [unwired: 2 in, 2 out]
            n791 = property on="Z Scan OK" class="Bool"("DisabledEnum"=T2."Enabled" ("Disabled")) -> ()  [unwired: 2 in, 2 out]
          }
        }
        n792 = property on="Scan Go" class="Bool"("DisabledEnum"=T2."Disabled and Grayed Out" ("Disabled")) -> ()  [unwired: 2 in, 2 out]
        n793 = property on="Scan Cancel" class="Bool"("DisabledEnum"=T2."Disabled and Grayed Out" ("Disabled")) -> ()  [unwired: 2 in, 2 out]
      }
      event "Scan Go": Mouse Up {
        n794 = event-data() -> ()  [unwired: 1 in, 7 out]
        n795 = flat-sequence {
          tunnel: w1371 -> [w1385]
          tunnel: w1370 -> [w1386]
          tunnel: w1369 -> [w1383]
          tunnel: w1368 -> [w1384]
          tunnel: w1367 -> [w1382]
          tunnel: w1366 -> [w1381]
          tunnel: [w1380] -> w1359
          tunnel: [w1379] -> w1357
          tunnel: [w1378] -> w1355
          tunnel: [w1377] -> w1353
          tunnel: [w1376] -> w1351
          tunnel: [w1375] -> w1349
          tunnel: [w1374] -> w1347
          tunnel: [w1373] -> w1346
          tunnel: [w1372] -> w1345
          tunnel: w1359 -> [w1428]
          tunnel: [w1427] -> w1358
          tunnel: w1357 -> [w1426]
          tunnel: [w1425] -> w1356
          tunnel: w1355 -> [w1424]
          tunnel: [w1423] -> w1354
          tunnel: w1353 -> [w1422]
          tunnel: [w1421] -> w1352
          tunnel: w1351 -> [w1420]
          tunnel: [w1419] -> w1350
          tunnel: w1349 -> [w1417]
          tunnel: [w1418] -> w1348
          tunnel: w1347 -> [w1416]
          tunnel: w1346 -> [w1415]
          tunnel: w1345 -> [w1414]
          tunnel: [w1454] -> w1365
          tunnel: [w1453] -> w1364
          tunnel: [w1452] -> w1363
          tunnel: [w1451] -> w1362
          tunnel: [w1456] -> w1361
          tunnel: [w1455] -> w1360
          tunnel: w1358 -> [w1456]
          tunnel: w1356 -> [w1455]
          tunnel: w1354 -> [w1454]
          tunnel: w1352 -> [w1453]
          tunnel: w1350 -> [w1452]
          tunnel: w1348 -> [w1451]
          frame #0 {
            n796 = property on="X Scan" class="Bool (strict)"() -> ("Value"=w1372:bool)  [unwired: 2 in, 2 out]
            n797 = property on="Y Scan" class="Bool (strict)"() -> ("Value"=w1373:bool)  [unwired: 2 in, 2 out]
            n798 = property on="Z Scan" class="Bool (strict)"() -> ("Value"=w1374:bool)  [unwired: 2 in, 2 out]
            n799 = case shown="True" w1372 {
              tunnel: w1386 -> [w1397 w1401]
              tunnel: [w1397 w1400] -> w1379
              tunnel: w1385 -> [w1396 w1399]
              tunnel: [w1396 w1398] -> w1380
              frame False {
              }
              frame True {
                n800 = property on="X Scan Length SP steps" class="DigNum (strict)"() -> ("Value"=w1402:i32)  [unwired: 2 in, 2 out]
                n801 = Number To Decimal String(number=w1402) -> (decimal integer string=w1403:string)  [unwired: 1 in]
                n802 = call "Applied Send Command.vi"("error in (no error)"=w1401, "Extra"=w1403, "Command"=T1."Distance or Position", "VISA resource name"=w1399) -> ("error out"=w1400:errorcluster, "VISA resource name out"=w1398:refnum<visa-resource-name>)  [unwired: 3 in, 1 out]
              }
            }
            n803 = case shown="True" w1373 {
              tunnel: w1383 -> [w1406 w1411]
              tunnel: w1384 -> [w1405 w1410]
              tunnel: [w1405 w1407] -> w1377
              tunnel: [w1406 w1408] -> w1378
              frame False {
              }
              frame True {
                n804 = property on="Y Scan Length SP steps" class="DigNum (strict)"() -> ("Value"=w1409:i32)  [unwired: 2 in, 2 out]
                n805 = Number To Decimal String(number=w1409) -> (decimal integer string=w1412:string)  [unwired: 1 in]
                n806 = call "Applied Send Command.vi"("error in (no error)"=w1410, "Extra"=w1412, "Command"=T1."Distance or Position", "VISA resource name"=w1411) -> ("error out"=w1407:errorcluster, "VISA resource name out"=w1408:refnum<visa-resource-name>)  [unwired: 3 in, 1 out]
              }
            }
            n807 = case shown="True" w1374 {
              tunnel: w1382 -> [w1388 w1392]
              tunnel: [w1388 w1391] -> w1376
              tunnel: [w1387 w1390] -> w1375
              tunnel: w1381 -> [w1387 w1389]
              frame False {
              }
              frame True {
                n808 = property on="Z Scan Length SP steps" class="DigNum (strict)"() -> ("Value"=w1393:i32)  [unwired: 2 in, 2 out]
                n809 = Number To Decimal String(number=w1393) -> (decimal integer string=w1394:string)  [unwired: 1 in]
                n810 = call "Applied Send Command.vi"("error in (no error)"=w1389, "Extra"=w1394, "Command"=T1."Distance or Position", "VISA resource name"=w1392) -> ("error out"=w1390:errorcluster, "VISA resource name out"=w1391:refnum<visa-resource-name>)  [unwired: 3 in, 1 out]
              }
            }
          }
          frame #1 {
            n811 = case shown="True" w1414 {
              tunnel: w1428 -> [w1444 w1448]
              tunnel: [w1444 w1447] -> w1427
              tunnel: w1426 -> [w1443 w1446]
              tunnel: [w1443 w1445] -> w1425
              frame False {
              }
              frame True {
                n812 = call "Applied Send Command.vi"("error in (no error)"=w1446, "Command"=T1."Feed to Length", "VISA resource name"=w1448) -> ("error out"=w1445:errorcluster, "VISA resource name out"=w1447:refnum<visa-resource-name>)  [unwired: 4 in, 1 out]
              }
            }
            n813 = case shown="True" w1415 {
              tunnel: w1424 -> [w1437 w1441]
              tunnel: [w1437 w1440] -> w1423
              tunnel: w1422 -> [w1436 w1439]
              tunnel: [w1436 w1438] -> w1421
              frame False {
              }
              frame True {
                n814 = call "Applied Send Command.vi"("error in (no error)"=w1439, "Command"=T1."Feed to Length", "VISA resource name"=w1441) -> ("error out"=w1438:errorcluster, "VISA resource name out"=w1440:refnum<visa-resource-name>)  [unwired: 4 in, 1 out]
              }
            }
            n815 = case shown="False" w1416 {
              tunnel: w1420 -> [w1430 w1434]
              tunnel: [w1430 w1433] -> w1419
              tunnel: [w1429 w1432] -> w1418
              tunnel: w1417 -> [w1429 w1431]
              frame False {
              }
              frame True {
                n816 = call "Applied Send Command.vi"("error in (no error)"=w1431, "Command"=T1."Feed to Length", "VISA resource name"=w1434) -> ("error out"=w1432:errorcluster, "VISA resource name out"=w1433:refnum<visa-resource-name>)  [unwired: 4 in, 1 out]
              }
            }
          }
          frame #2 {
            (unwired) FALSE ("Slew Ready 2")
            n817 = call "Time Delay7"("Delay Time (s)"=0.1) -> ()  [unwired: 10 in, 1 out]
            n818 = property on="Z Scan" class="Bool (strict)"("Val(Sgnl)"=FALSE ("Slew Ready 2")) -> ()  [unwired: 2 in, 2 out]
            n819 = property on="X Scan" class="Bool (strict)"("Val(Sgnl)"=FALSE ("Slew Ready 2")) -> ()  [unwired: 2 in, 2 out]
            n820 = property on="Y Scan" class="Bool (strict)"("Val(Sgnl)"=FALSE ("Slew Ready 2")) -> ()  [unwired: 2 in, 2 out]
            n821 = property on="Z Scan Velocity SP steps/sec" class="DigNum (strict)"("DisabledEnum"=T2."Enabled" ("Disabled")) -> ()  [unwired: 2 in, 2 out]
            n822 = property on="X Scan Length SP steps" class="DigNum (strict)"("DisabledEnum"=T2."Enabled" ("Disabled")) -> ()  [unwired: 2 in, 2 out]
            n823 = property on="Y Scan Selocity SP steps/sec" class="DigNum (strict)"("DisabledEnum"=T2."Enabled" ("Disabled")) -> ()  [unwired: 2 in, 2 out]
            n824 = property on="Z Scan Length SP steps" class="DigNum (strict)"("DisabledEnum"=T2."Enabled" ("Disabled")) -> ()  [unwired: 2 in, 2 out]
            n825 = property on="Y Scan Length SP steps" class="DigNum (strict)"("DisabledEnum"=T2."Enabled" ("Disabled")) -> ()  [unwired: 2 in, 2 out]
            n826 = property on="X Scan Velocity SP steps/sec" class="DigNum (strict)"("DisabledEnum"=T2."Enabled" ("Disabled")) -> ()  [unwired: 2 in, 2 out]
            n827 = property on="Scan Go" class="Bool"("DisabledEnum"=T2."Disabled and Grayed Out" ("Disabled")) -> ()  [unwired: 2 in, 2 out]
            n828 = property on="Scan Cancel" class="Bool"("DisabledEnum"=T2."Disabled and Grayed Out" ("Disabled")) -> ()  [unwired: 2 in, 2 out]
          }
        }
      }
      event "Reset": Mouse Down {
        n829 = event-data() -> ()  [unwired: 1 in, 7 out]
        n830 = flat-sequence {
          tunnel: [w1487] -> w1473
          tunnel: w1474 -> [w1489]
          tunnel: [w1488] -> w1472
          tunnel: w1475 -> [w1490]
          frame #0 {
            n831 = property on="Reset X Motor Steps" class="DigNum (strict)"() -> ("Value"=w1493:i32)  [unwired: 2 in, 2 out]
            n832 = Number To Decimal String(number=w1493) -> (decimal integer string=w1491:string)  [unwired: 1 in]
            n833 = call "Applied Send Command.vi"("error in (no error)"=w1489, "Extra"=w1491, "Command"=T1."Set ABS Position", "VISA resource name"=w1490) -> ("error out"=w1488:errorcluster, "VISA resource name out"=w1487:refnum<visa-resource-name>)  [unwired: 3 in, 1 out]
          }
        }
        n834 = flat-sequence {
          tunnel: w1479 -> [w1498]
          tunnel: w1478 -> [w1495]
          tunnel: [w1497] -> w1477
          tunnel: [w1496] -> w1476
          frame #0 {
            n835 = property on="Reset Y Motor Steps" class="DigNum (strict)"() -> ("Value"=w1500:i32)  [unwired: 2 in, 2 out]
            n836 = Number To Decimal String(number=w1500) -> (decimal integer string=w1499:string)  [unwired: 1 in]
            n837 = call "Applied Send Command.vi"("error in (no error)"=w1495, "Extra"=w1499, "Command"=T1."Set ABS Position", "VISA resource name"=w1498) -> ("error out"=w1496:errorcluster, "VISA resource name out"=w1497:refnum<visa-resource-name>)  [unwired: 3 in, 1 out]
          }
        }
        n838 = flat-sequence {
          tunnel: [w1485] -> w1469
          tunnel: [w1484] -> w1468
          tunnel: w1471 -> [w1482]
          tunnel: w1470 -> [w1483]
          frame #0 {
            n839 = property on="Reset Z Motor Steps" class="DigNum (strict)"() -> ("Value"=w1486:i32)  [unwired: 2 in, 2 out]
            n840 = Number To Decimal String(number=w1486) -> (decimal integer string=w1480:string)  [unwired: 1 in]
            n841 = call "Applied Send Command.vi"("error in (no error)"=w1483, "Extra"=w1480, "Command"=T1."Set ABS Position", "VISA resource name"=w1482) -> ("error out"=w1484:errorcluster, "VISA resource name out"=w1485:refnum<visa-resource-name>)  [unwired: 3 in, 1 out]
          }
        }
      }
    }
    n842 = case shown="True" "Delete Button" {
      tunnel: w287 -> [_ w310]
      frame False {
      }
      frame True {
        n843 = property on="Preset positions" class="Ring (strict)"() -> ("Value"=w308:i32)  [unwired: 2 in, 2 out]
        n844 = Delete From Array(array=w310, index=w308) -> (array with subset deleted=w309:string[])  [unwired: 1 in, 1 out]
        n845 = property on="Presets" class="Arr (strict)"() -> ("Value"=w307:i32[][])  [unwired: 2 in, 2 out]
        n846 = property on="Preset positions" class="Ring (strict)"("Strings []"=w309) -> ()  [unwired: 2 in, 2 out]
        n847 = Delete From Array(array=w307, index (row)=w308) -> (array with subset deleted=w306:i32[][])  [unwired: 2 in, 1 out]
        n848 = property on="Presets" class="Arr (strict)"("Val(Sgnl)"=w306) -> ()  [unwired: 2 in, 2 out]
      }
    }
    n849 = case shown="True" "Set Button" {
      tunnel: "Preset positions" -> [_ w326]
      frame False {
      }
      frame True {
        n850 = property on="Presets" class="Arr (strict)"() -> ("Value"=w323:i32[][])  [unwired: 2 in, 2 out]
        n851 = Index Array(array=w323, index (row)=w326) -> (element=w325:i32[])  [unwired: 1 in]
        n852 = Array To Cluster(array=w325) -> (cluster=w324:T4)
        n853 = Unbundle(w324) -> ("Value[0]"=w322:i32, "Value[1]"=w321:i32, "Value[2]"=w320:i32)  [unwired: 6 out]
        n854 = property on="X Step SP" class="DigNum (strict)"("Val(Sgnl)"=w322) -> ()  [unwired: 2 in, 2 out]
        n855 = property on="Y Step SP" class="DigNum (strict)"("Val(Sgnl)"=w321) -> ()  [unwired: 2 in, 2 out]
        n856 = property on="Z Step SP" class="DigNum (strict)"("Val(Sgnl)"=w320) -> ()  [unwired: 2 in, 2 out]
      }
    }
    n857 = case shown="True" "Add Button" {
      tunnel: w287 -> [_ w319]
      frame False {
      }
      frame True {
        n858 = property on="X Step PV" class="DigNum (strict)"() -> ("Value"=w314:i32)  [unwired: 2 in, 2 out]
        n859 = property on="Y Step PV" class="DigNum (strict)"() -> ("Value"=w313:i32)  [unwired: 2 in, 2 out]
        n860 = property on="Z Step PV" class="DigNum (strict)"() -> ("Value"=w312:i32)  [unwired: 2 in, 2 out]
        n861 = Build Array(w314, w313, w312) -> (w317:i32[])
        n862 = Build Array (concatenate)(w319, "String") -> (w318:string[])
        n863 = property on="Preset positions" class="Ring (strict)"("Strings []"=w318) -> ()  [unwired: 2 in, 2 out]
        n864 = property on="Presets" class="Arr (strict)"() -> ("Value"=w316:i32[][])  [unwired: 2 in, 2 out]
        n865 = Build Array (concatenate)(w316, w317) -> (w311:i32[][])
        n866 = property on="Presets" class="Arr (strict)"("Val(Sgnl)"=w311) -> ()  [unwired: 2 in, 2 out]
      }
    }
  }
  n867 = flat-sequence {
    tunnel: w55 -> [w1502]
    tunnel: w54 -> [w1501]
    tunnel: [w1513] -> w39
    frame #0 {
      # "GET CURRENT POSITION"
      n868 = call "Applied Send Command.vi"("error in (no error)"=w1501, "Extra"="", "Command"=T1."Immediate Position?", "VISA resource name"=w1502) -> ("error out"=w1503:errorcluster, "read buffer"=w1508:string, "VISA resource name out"=w1504:refnum<visa-resource-name>)  [unwired: 3 in]
      n869 = call "Applied Send Command.vi"("error in (no error)"=w1503, "Command"=T1."Stop & Kill Buffer", "VISA resource name"=w1504) -> ("error out"=w1510:errorcluster, "VISA resource name out"=w1511:refnum<visa-resource-name>)  [unwired: 4 in, 1 out]
      n870 = Hexadecimal String To Number(string=w1508, offset=3) -> (number=w1505:u32)  [unwired: 1 in, 1 out]
      n871 = VISA Close(VISA resource name=w1511, error in (no error)=w1510) -> ()  [unwired: 1 out]
      n872 = To Long Integer(number=w1505) -> (32bit integer=w1513:i32)
    }
  }
  n873 = flat-sequence {
    tunnel: w41 -> [w1516]
    tunnel: w40 -> [w1515]
    tunnel: [w1514] -> w38
    frame #0 {
      # "GET CURRENT POSITION"
      n874 = call "Applied Send Command.vi"("error in (no error)"=w1515, "Extra"="", "Command"=T1."Immediate Position?", "VISA resource name"=w1516) -> ("error out"=w1517:errorcluster, "read buffer"=w1522:string, "VISA resource name out"=w1518:refnum<visa-resource-name>)  [unwired: 3 in]
      n875 = call "Applied Send Command.vi"("error in (no error)"=w1517, "Command"=T1."Stop & Kill Buffer", "VISA resource name"=w1518) -> ("error out"=w1524:errorcluster, "VISA resource name out"=w1525:refnum<visa-resource-name>)  [unwired: 4 in, 1 out]
      n876 = Hexadecimal String To Number(string=w1522, offset=3) -> (number=w1519:u32)  [unwired: 1 in, 1 out]
      n877 = VISA Close(VISA resource name=w1525, error in (no error)=w1524) -> ()  [unwired: 1 out]
      n878 = To Long Integer(number=w1519) -> (32bit integer=w1514:i32)
    }
  }
  n879 = flat-sequence {
    tunnel: w43 -> [w1528]
    tunnel: w42 -> [w1527]
    tunnel: [w1529] -> w37
    frame #0 {
      # "GET CURRENT POSITION"
      n880 = call "Applied Send Command.vi"("error in (no error)"=w1527, "Extra"="", "Command"=T1."Immediate Position?", "VISA resource name"=w1528) -> ("error out"=w1530:errorcluster, "read buffer"=w1535:string, "VISA resource name out"=w1531:refnum<visa-resource-name>)  [unwired: 3 in]
      n881 = call "Applied Send Command.vi"("error in (no error)"=w1530, "Command"=T1."Stop & Kill Buffer", "VISA resource name"=w1531) -> ("error out"=w1537:errorcluster, "VISA resource name out"=w1538:refnum<visa-resource-name>)  [unwired: 4 in, 1 out]
      n882 = Hexadecimal String To Number(string=w1535, offset=3) -> (number=w1532:u32)  [unwired: 1 in, 1 out]
      n883 = VISA Close(VISA resource name=w1538, error in (no error)=w1537) -> ()  [unwired: 1 out]
      n884 = To Long Integer(number=w1532) -> (32bit integer=w1529:i32)
    }
  }
  n885 = flat-sequence {
    tunnel: w39 -> [w1544]
    tunnel: w38 -> [w1543]
    tunnel: w37 -> [w1542]
    frame #0 {
      n886 = Build Array(w1544, w1543, w1542) -> (w1540:i32[])
      n887 = call-poly <vilib>:"Write To Spreadsheet File.vi"("1D data"=w1540, "file path (dialog if empty)"=path "S:/SSE/SCL2/POS.TXT") -> ()  [unwired: 6 in, 1 out]
    }
    frame #1 {
      n888 = property on="Presets" class="Arr (strict)"() -> ("Value"=w1551:i32[][])  [unwired: 2 in, 2 out]
      n889 = property on="Preset positions" class="Ring (strict)"() -> ("Strings []"=w1547:string[])  [unwired: 2 in, 2 out]
      n890 = Number To Decimal String(number=w1551) -> (decimal integer string=w1545:string[][])  [unwired: 1 in]
      n891 = Transpose 2D Array(2D array=w1545) -> (transposed array=w1546:string[][])
      n892 = Build Array (concatenate)(w1547, w1546) -> (w1548:string[][])
      n893 = Transpose 2D Array(2D array=w1548) -> (transposed array=w1549:string[][])
      n894 = call-poly <vilib>:"Write To Spreadsheet File.vi"("2D data"=w1549, "file path (dialog if empty)"=path "S:/SSE/SCL2/PRESET.TXT") -> ()  [unwired: 6 in, 1 out]
    }
  }
